vi "37YY250X-1 Phillips DXR.vi"() -> ()   [LabVIEW 2013]
uses:
  <vilib>/Instr/_visa.llb/VISA Configure Serial Port (Instr).vi
panel:
  in  "enumPart":T1(ring)
  in  "Serial Port":refnum<visa-resource-name>
  out "String":string
  out "bDomeClosed":bool
  out "SW VER":string
  out "Employee ID":string
  out "dlbLED":dbl[](array[numeric])
  out "Serial Out 2":i32[](array[numeric])
  out "dlbAllLEDs":dbl
  out "bPassFail":bool
  out "TIMER":dbl
  in  "btnStart":bool
  out "bKeys":bool
  out "bLEDs":bool
  in  "btnExit":bool
  out "Cluster":T2
  out "Serial Out":i32[](array[numeric])
  in  "btnStop":bool
  out "Serial In":u8[](array[numeric])=[165, 1, 31, 32] format="%.0x"
  out "Boolean":bool
  # "Serial Data\nByte 0 Sync\nByte 1 CMD\nByte 2 PORT DATA\nByte 3 BitMask\nByte 4 KeyMap"
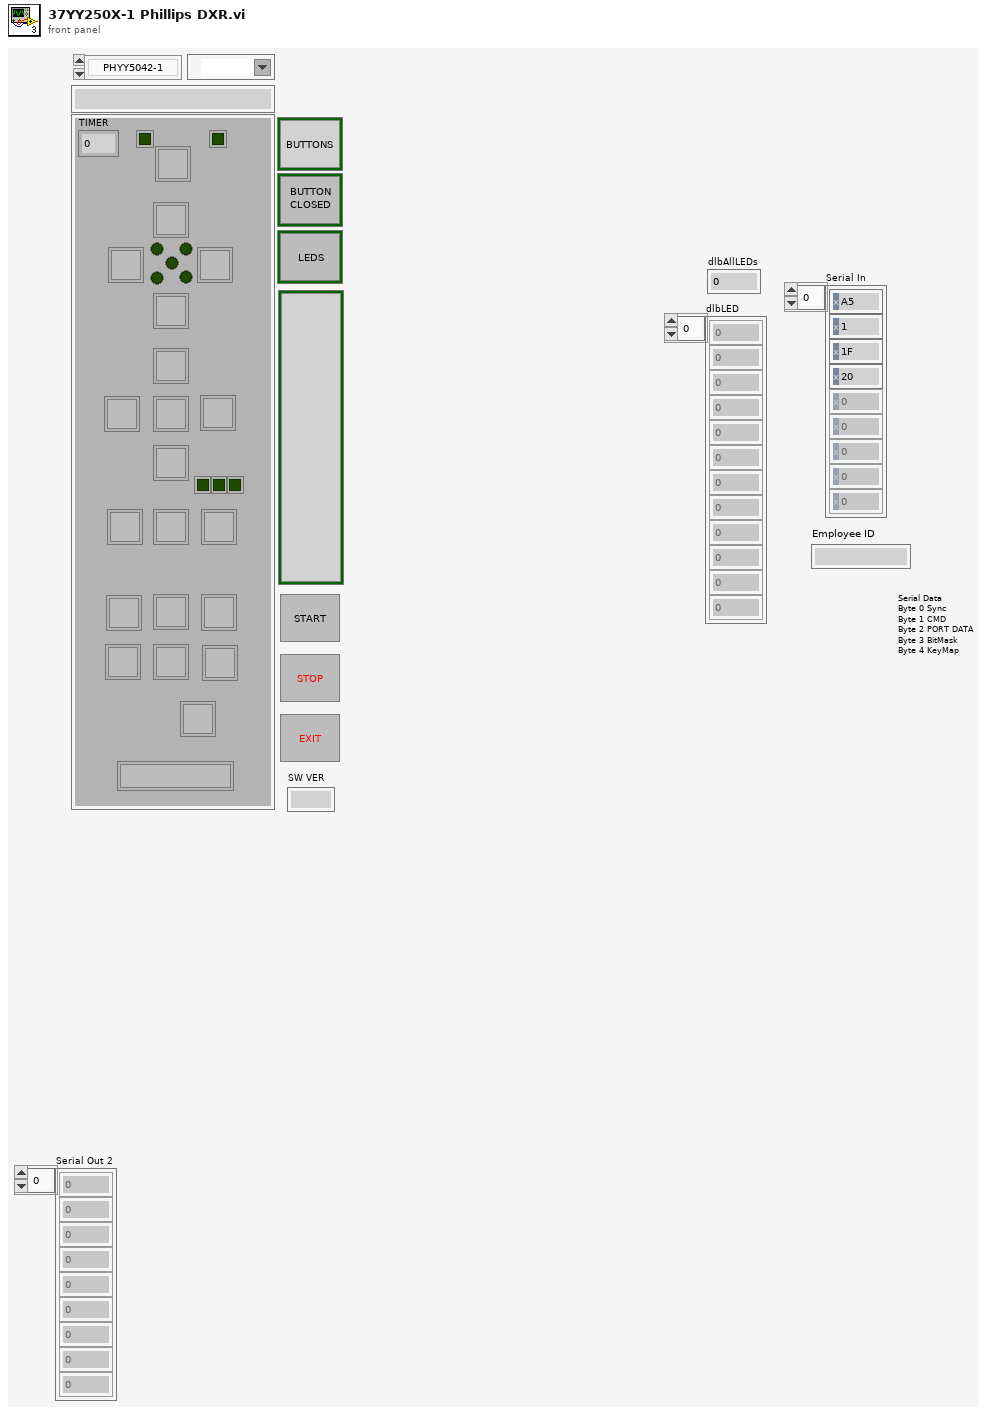
[diagram p1: front panel]
types:
  T1 = enum16{"PHYY5042-1", "PHYY5043-1", "PHYY5037-1", "PHYY5037-2", "PHYY5071-1", "PHYY5071-2", "PHYY5110-1", "PHYY5110-2"}
  T2 = cluster{"bLed 0":bool, "bLed 1":bool, "bLed 2":bool, "bLed 3":bool, "bLed 4":bool, "bLed 5":bool, "bLed 6":bool, "bLed 7":bool, "bLed 8":bool, "bLed 9":bool, "DS 1":bool, "DS 2":bool, "DS 3":bool, "DS 4":bool, "DS 5":bool, "DS 6":bool, "DS 7":bool, "DS 8":bool, "DS 9":bool, "DS 10":bool, "DS 11":bool, "DS 12":bool, "DS 13":bool, "DS 14":bool, "DS 15":bool, "DS 16":bool, "DS 17":bool, "DS 18":bool, "DS 19":bool, "DS 20":bool, "DS 21":bool, "bFalseImage":bool, "bFalseImage 2":bool, "bIcon":bool, "bIcon 2":bool, "Boolean":bool, "Boolean 2":bool, "Boolean 3":bool}
  T3 = enum8{"Enabled", "Disabled", "Disabled and Grayed Out"}
  T4 = cluster{"LOG_DIRECTORY":string, "LOG_FILE":string, "Part Number":string[], "Base Part Number":string[]}
  T5 = enum16{"SET DEFAULTS", "ENABLE POWER", "SCAN FOR CLOSED KEYS", "KEY TEST", "LED TEST", "DISABLE POWER", "TEST END"}
  T6 = cluster{"dlbLED":dbl[], "dlbAllLEDs":dbl, "Pass/Fail":bool, "Keys":bool, "LEDS":bool, "Employee ID":string, "Part Number":string, "SW Version":string}
  T7 = enum32{"invalid app kind", "Development System", "Run Time System", "Student Edition", "Embedded LabVIEW", "Evaluation", "Custom"}
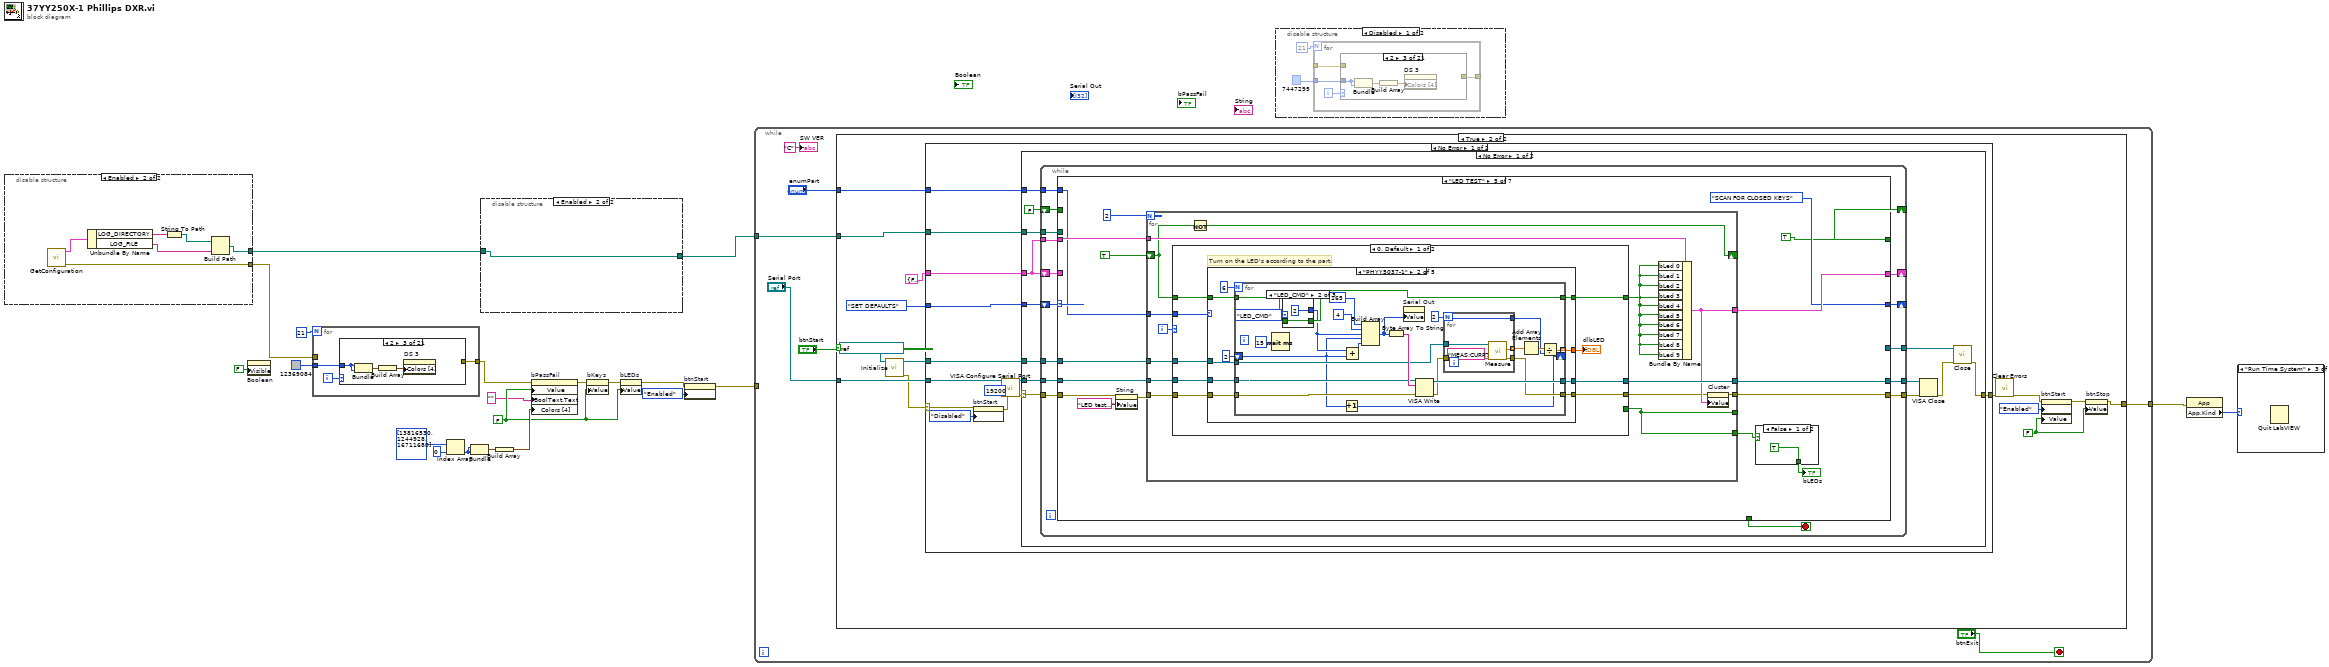
[diagram p0: block diagram]
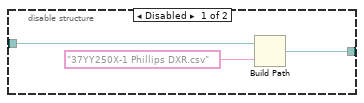
[diagram p8: hidden frame]
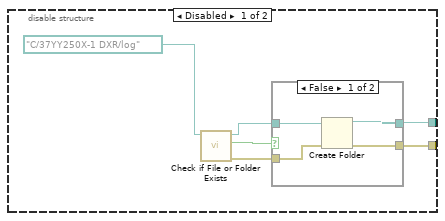
[diagram p9: hidden frame]
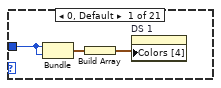
[diagram p11: hidden frame]
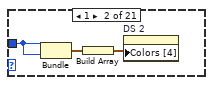
[diagram p12: hidden frame]
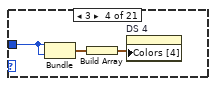
[diagram p13: hidden frame]
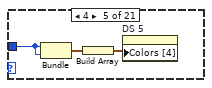
[diagram p14: hidden frame]
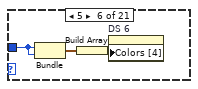
[diagram p15: hidden frame]
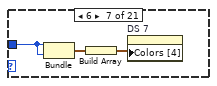
[diagram p16: hidden frame]
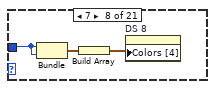
[diagram p17: hidden frame]
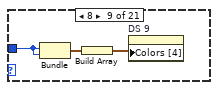
[diagram p18: hidden frame]
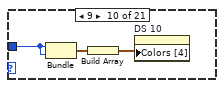
[diagram p19: hidden frame]
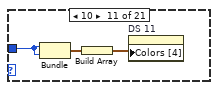
[diagram p20: hidden frame]
diagram:
  w15 = FALSE ("bKeys")
  n1 = disable-structure shown="Enabled" {
    disable-tunnel: [w26 w36] -> w5
    disable-tunnel: [w23 w38] -> w4
    frame Disabled {
      n2 = call <vilib>:"Check if File or Folder Exists.vi"("path"=path "C:/37YY250X-1 DXR/log" ("file path (dialog if empty)")) -> ("error out"=w24:errorcluster, "file or folder exists?"=w27:bool, "dup path"=w25:path)  [unwired: 8 in]
      n3 = case shown="False" w27 {
        tunnel: [w30 w32] -> w26
        tunnel: w25 -> [w31 w32]
        tunnel: w24 -> [w29 _]
        tunnel: [w28 _] -> w23
        frame False {
          n4 = Create Folder(path (use dialog)=w31, error in=w29) -> (created path=w30:path, error out=w28:errorcluster)  [unwired: 1 in, 1 out]
        }
        frame True {
        }
      }
    }
    frame Enabled {
      n5 = call "GetConfiguration.vi"() -> ("error out"=w38:errorcluster, "Cluster"=w37:T4)  [unwired: 9 in, 1 out]
      n6 = Unbundle By Name(w37) -> ("LOG_DIRECTORY"=w35:string, "LOG_FILE"=w33:string)
      n7 = String To Path(string=w35) -> (path=w34:path)
      n8 = Build Path(base path=w34, name or relative path=w33) -> (appended path=w36:path)
    }
  }
  n9 = property on="Boolean" class="Bool (strict)"("Visible"=FALSE) -> ()  [unwired: 2 in, 2 out]
  n10 = for {
    N: 21 -> [_]
    tunnel: u32 12369084 -> [w40]
    tunnel: [w39] -> w7
    tunnel: w4 -> [_]
    i -> [w41]
    n11 = case shown="2" w41 {
      tunnel: w40 -> [w42 w45 w48 w51 w54 w57 w60 w63 w66 w69 w72 w75 w78 w81 w84 w87 w90 w93 w96 w99 w103]
      tunnel: [_ _ _ _ _ _ _ _ _ _ _ _ _ _ _ _ _ _ _ _ w102] -> w39
      frame 0, Default {
        n12 = Bundle(w42, w42) -> (w44:cluster{u32, u32})  [unwired: 1 in]
        n13 = Build Array(w44) -> (w43:cluster{u32, u32}[])
        n14 = property on="DS 1" class="Bool (strict)"("Colors [4]"=w43) -> ()  [unwired: 2 in, 2 out]
      }
      frame 1 {
        n15 = Bundle(w45, w45) -> (w47:cluster{u32, u32})  [unwired: 1 in]
        n16 = Build Array(w47) -> (w46:cluster{u32, u32}[])
        n17 = property on="DS 2" class="Bool (strict)"("Colors [4]"=w46) -> ()  [unwired: 2 in, 2 out]
      }
      frame 2 {
        n18 = Bundle(w48, w48) -> (w50:cluster{u32, u32})  [unwired: 1 in]
        n19 = Build Array(w50) -> (w49:cluster{u32, u32}[])
        n20 = property on="DS 3" class="Bool (strict)"("Colors [4]"=w49) -> ()  [unwired: 2 in, 2 out]
      }
      frame 3 {
        n21 = Bundle(w51, w51) -> (w52:cluster{u32, u32})  [unwired: 1 in]
        n22 = Build Array(w52) -> (w53:cluster{u32, u32}[])
        n23 = property on="DS 4" class="Bool (strict)"("Colors [4]"=w53) -> ()  [unwired: 2 in, 2 out]
      }
      frame 4 {
        n24 = Bundle(w54, w54) -> (w56:cluster{u32, u32})  [unwired: 1 in]
        n25 = Build Array(w56) -> (w55:cluster{u32, u32}[])
        n26 = property on="DS 5" class="Bool (strict)"("Colors [4]"=w55) -> ()  [unwired: 2 in, 2 out]
      }
      frame 5 {
        n27 = Bundle(w57, w57) -> (w59:cluster{u32, u32})  [unwired: 1 in]
        n28 = Build Array(w59) -> (w58:cluster{u32, u32}[])
        n29 = property on="DS 6" class="Bool (strict)"("Colors [4]"=w58) -> ()  [unwired: 2 in, 2 out]
      }
      frame 6 {
        n30 = Bundle(w60, w60) -> (w62:cluster{u32, u32})  [unwired: 1 in]
        n31 = Build Array(w62) -> (w61:cluster{u32, u32}[])
        n32 = property on="DS 7" class="Bool (strict)"("Colors [4]"=w61) -> ()  [unwired: 2 in, 2 out]
      }
      frame 7 {
        n33 = Bundle(w63, w63) -> (w65:cluster{u32, u32})  [unwired: 1 in]
        n34 = Build Array(w65) -> (w64:cluster{u32, u32}[])
        n35 = property on="DS 8" class="Bool (strict)"("Colors [4]"=w64) -> ()  [unwired: 2 in, 2 out]
      }
      frame 8 {
        n36 = Bundle(w66, w66) -> (w68:cluster{u32, u32})  [unwired: 1 in]
        n37 = Build Array(w68) -> (w67:cluster{u32, u32}[])
        n38 = property on="DS 9" class="Bool (strict)"("Colors [4]"=w67) -> ()  [unwired: 2 in, 2 out]
      }
      frame 9 {
        n39 = Bundle(w69, w69) -> (w71:cluster{u32, u32})  [unwired: 1 in]
        n40 = Build Array(w71) -> (w70:cluster{u32, u32}[])
        n41 = property on="DS 10" class="Bool (strict)"("Colors [4]"=w70) -> ()  [unwired: 2 in, 2 out]
      }
      frame 10 {
        n42 = Bundle(w72, w72) -> (w74:cluster{u32, u32})  [unwired: 1 in]
        n43 = Build Array(w74) -> (w73:cluster{u32, u32}[])
        n44 = property on="DS 11" class="Bool (strict)"("Colors [4]"=w73) -> ()  [unwired: 2 in, 2 out]
      }
      frame 11 {
        n45 = Bundle(w75, w75) -> (w76:cluster{u32, u32})  [unwired: 1 in]
        n46 = Build Array(w76) -> (w77:cluster{u32, u32}[])
        n47 = property on="DS 12" class="Bool (strict)"("Colors [4]"=w77) -> ()  [unwired: 2 in, 2 out]
      }
      frame 12 {
        n48 = Bundle(w78, w78) -> (w80:cluster{u32, u32})  [unwired: 1 in]
        n49 = Build Array(w80) -> (w79:cluster{u32, u32}[])
        n50 = property on="DS 13" class="Bool (strict)"("Colors [4]"=w79) -> ()  [unwired: 2 in, 2 out]
      }
      frame 13 {
        n51 = Bundle(w81, w81) -> (w83:cluster{u32, u32})  [unwired: 1 in]
        n52 = Build Array(w83) -> (w82:cluster{u32, u32}[])
        n53 = property on="DS 14" class="Bool (strict)"("Colors [4]"=w82) -> ()  [unwired: 2 in, 2 out]
      }
      frame 14 {
        n54 = Bundle(w84, w84) -> (w86:cluster{u32, u32})  [unwired: 1 in]
        n55 = Build Array(w86) -> (w85:cluster{u32, u32}[])
        n56 = property on="DS 15" class="Bool (strict)"("Colors [4]"=w85) -> ()  [unwired: 2 in, 2 out]
      }
      frame 15 {
        n57 = Bundle(w87, w87) -> (w89:cluster{u32, u32})  [unwired: 1 in]
        n58 = Build Array(w89) -> (w88:cluster{u32, u32}[])
        n59 = property on="DS 16" class="Bool (strict)"("Colors [4]"=w88) -> ()  [unwired: 2 in, 2 out]
      }
      frame 16 {
        n60 = Bundle(w90, w90) -> (w92:cluster{u32, u32})  [unwired: 1 in]
        n61 = Build Array(w92) -> (w91:cluster{u32, u32}[])
        n62 = property on="DS 17" class="Bool (strict)"("Colors [4]"=w91) -> ()  [unwired: 2 in, 2 out]
      }
      frame 17 {
        n63 = Bundle(w93, w93) -> (w95:cluster{u32, u32})  [unwired: 1 in]
        n64 = Build Array(w95) -> (w94:cluster{u32, u32}[])
        n65 = property on="DS 18" class="Bool (strict)"("Colors [4]"=w94) -> ()  [unwired: 2 in, 2 out]
      }
      frame 18 {
        n66 = Bundle(w96, w96) -> (w98:cluster{u32, u32})  [unwired: 1 in]
        n67 = Build Array(w98) -> (w97:cluster{u32, u32}[])
        n68 = property on="DS 19" class="Bool (strict)"("Colors [4]"=w97) -> ()  [unwired: 2 in, 2 out]
      }
      frame 19 {
        n69 = Bundle(w99, w99) -> (w101:cluster{u32, u32})  [unwired: 1 in]
        n70 = Build Array(w101) -> (w100:cluster{u32, u32}[])
        n71 = property on="DS 20" class="Bool (strict)"("Colors [4]"=w100) -> ()  [unwired: 2 in, 2 out]
      }
      frame 20 {
        n72 = Bundle(w103, w103) -> (w105:cluster{u32, u32})  [unwired: 1 in]
        n73 = Build Array(w105) -> (w104:cluster{u32, u32}[])
        n74 = property on="DS 21" class="Bool (strict)"("Colors [4]"=w104) -> (error out=w102:errorcluster)  [unwired: 2 in, 1 out]
      }
    }
  }
  n75 = Index Array(array=u32[] [13816530, 1244928, 16711680], index=0) -> (element=w18:u32)
  n76 = Bundle(w18, w18) -> (w19:cluster{u32, u32})  [unwired: 1 in]
  n77 = disable-structure shown="Enabled" {
    disable-tunnel: [w107 w109] -> w6
    disable-tunnel: w5 -> [w106 w109]
    frame Disabled {
      n78 = Build Path(base path=w106, name or relative path="37YY250X-1 Phillips DXR.csv") -> (appended path=w107:path)
    }
    frame Enabled {
    }
  }
  n79 = Build Array(w19) -> (w20:cluster{u32, u32}[])
  n80 = property on="bPassFail" class="Bool (strict)"(error in=w7, "Value"=w15, "BoolText.Text"="" ("Boolean Text.Text"), "Colors [4]"=w20) -> (error out=w13:errorcluster)  [unwired: 1 in, 1 out]
  n81 = property on="bKeys" class="Bool (strict)"(error in=w13, "Value"=w15) -> (error out=w12:errorcluster)  [unwired: 1 in, 1 out]
  n82 = property on="bLEDs" class="Bool (strict)"(error in=w12, "Value"=w15) -> (error out=w11:errorcluster)  [unwired: 1 in, 1 out]
  n83 = property on="btnStart" class="Bool (strict)"(error in=w11, "DisabledEnum"=T3."Enabled" ("Disabled")) -> (error out=w10:errorcluster)  [unwired: 1 in, 1 out]
  n84 = while {
    tunnel: [w115] -> w2
    tunnel: w10 -> [_]
    tunnel: w6 -> [w112]
    stop <- "btnExit" stop-if-true
    n85 = case shown="True" "btnStart" {
      tunnel: [_ w196] -> w115
      tunnel: w112 -> [w143 w192]
      tunnel: "Serial Port" -> [_ w191]
      tunnel: "enumPart" -> [w119 w189]
      frame False {
        n86 = case shown="\"PHYY5110-2\"" w119 {
          tunnel: [w148 w150 w152 w154 w155 w162 w174] -> w137
          tunnel: [w148 w150 w152 w154 w155 w163 w175] -> w136
          tunnel: [w148 w150 w152 w154 w155 w161 w173] -> w135
          tunnel: [w148 w150 w152 w154 w155 w164 w176] -> w134
          tunnel: [w148 w150 w152 w154 w155 w165 w177] -> w133
          tunnel: [w148 w150 w152 w154 w155 w166 w178] -> w132
          tunnel: [w148 w150 w152 w154 w155 w167 w179] -> w131
          tunnel: [w148 w150 w152 w154 w155 w158 w170] -> w130
          tunnel: [w148 w150 w152 w154 w155 w159 w171] -> w129
          tunnel: [w148 w150 w152 w154 w155 w159 w171] -> w128
          tunnel: [w148 w150 w152 w154 w155 w159 w171] -> w127
          tunnel: [w148 w150 w152 w154 w155 w159 w171] -> w126
          tunnel: [w148 _ _ _ _ w160 w172] -> w125
          tunnel: [w148 _ _ _ _ w160 w172] -> w124
          tunnel: [w148 _ _ _ _ w160 w172] -> w123
          tunnel: [w148 _ _ _ _ _ _] -> w122
          tunnel: [w148 w150 w152 w154 w155 w168 w180] -> w121
          tunnel: [FALSE TRUE TRUE w154 TRUE w160 w172] -> w120
          tunnel: [w148 w150 w152 w154 w155 w159 w171] -> w118
          tunnel: [_ _ _ _ _ TRUE TRUE] -> w117
          frame "PHYY5042-1", Default {
            w148 = TRUE
          }
          frame "PHYY5037-1" {
            w150 = FALSE
          }
          frame "PHYY5071-1" {
            w152 = FALSE
          }
          frame "PHYY5071-2" {
            w154 = TRUE
          }
          frame "PHYY5037-2" {
            w155 = FALSE
          }
          frame "PHYY5110-1" {
            w160 = FALSE
            w159 = TRUE
            n87 = Not(x=w159) -> (.not. x?=w158:bool)
            n88 = Not(x=w159) -> (.not. x?=w162:bool)
            n89 = Not(x=w159) -> (.not. x?=w163:bool)
            n90 = Not(x=w159) -> (.not. x?=w161:bool)
            n91 = Not(x=w159) -> (.not. x?=w164:bool)
            n92 = Not(x=w159) -> (.not. x?=w165:bool)
            n93 = Not(x=w159) -> (.not. x?=w166:bool)
            n94 = Not(x=w159) -> (.not. x?=w167:bool)
            n95 = Not(x=w159) -> (.not. x?=w168:bool)
          }
          frame "PHYY5110-2" {
            w172 = FALSE
            w171 = TRUE
            n96 = Not(x=w171) -> (.not. x?=w170:bool)
            n97 = Not(x=w171) -> (.not. x?=w174:bool)
            n98 = Not(x=w171) -> (.not. x?=w175:bool)
            n99 = Not(x=w171) -> (.not. x?=w173:bool)
            n100 = Not(x=w171) -> (.not. x?=w176:bool)
            n101 = Not(x=w171) -> (.not. x?=w177:bool)
            n102 = Not(x=w171) -> (.not. x?=w178:bool)
            n103 = Not(x=w171) -> (.not. x?=w179:bool)
            n104 = Not(x=w171) -> (.not. x?=w180:bool)
          }
        }
        n105 = property on="DS 15" class="Bool (strict)"("Visible"=w137) -> ()  [unwired: 2 in, 2 out]
        n106 = property on="DS 12" class="Bool (strict)"("Visible"=w136) -> ()  [unwired: 2 in, 2 out]
        n107 = property on="DS 14" class="Bool (strict)"("Visible"=w134) -> ()  [unwired: 2 in, 2 out]
        n108 = property on="DS 13" class="Bool (strict)"("Visible"=w135) -> ()  [unwired: 2 in, 2 out]
        n109 = property on="DS 8" class="Bool (strict)"("Visible"=w132) -> ()  [unwired: 2 in, 2 out]
        n110 = property on="DS 9" class="Bool (strict)"("Visible"=w131) -> ()  [unwired: 2 in, 2 out]
        n111 = property on="DS 11" class="Bool (strict)"("Visible"=w133) -> ()  [unwired: 2 in, 2 out]
        n112 = property on="DS 5" class="Bool (strict)"("Visible"=w129) -> ()  [unwired: 2 in, 2 out]
        n113 = property on="DS 10" class="Bool (strict)"("Visible"=w130) -> ()  [unwired: 2 in, 2 out]
        n114 = property on="DS 2" class="Bool (strict)"("Visible"=w128) -> ()  [unwired: 2 in, 2 out]
        n115 = property on="DS 7" class="Bool (strict)"("Visible"=w127) -> ()  [unwired: 2 in, 2 out]
        n116 = property on="DS 4" class="Bool (strict)"("Visible"=w126) -> ()  [unwired: 2 in, 2 out]
        n117 = property on="DS 1" class="Bool (strict)"("Visible"=w121) -> ()  [unwired: 2 in, 2 out]
        n118 = property on="DS 3" class="Bool (strict)"("Visible"=w118) -> ()  [unwired: 2 in, 2 out]
        n119 = property on="bFalseImage" class="Bool (strict)"("Visible"=w120) -> ()  [unwired: 2 in, 2 out]
        n120 = property on="bLed 1" class="Bool (strict)"("Visible"=w125) -> ()  [unwired: 2 in, 2 out]
        n121 = property on="bLed 7" class="Bool (strict)"("Visible"=w124) -> ()  [unwired: 2 in, 2 out]
        n122 = property on="bFalseImage 2" class="Bool (strict)"("Visible"=w120) -> ()  [unwired: 2 in, 2 out]
        n123 = property on="bLed 9" class="Bool (strict)"("Visible"=w122) -> ()  [unwired: 2 in, 2 out]
        n124 = property on="bLed 8" class="Bool (strict)"("Visible"=w123) -> ()  [unwired: 2 in, 2 out]
        n125 = property on="bIcon" class="Bool (strict)"("Visible"=w120) -> ()  [unwired: 2 in, 2 out]
        n126 = property on="bIcon 2" class="Bool (strict)"("Visible"=w120) -> ()  [unwired: 2 in, 2 out]
        n127 = property on="Boolean" class="Bool (strict)"("Visible"=w117) -> ()  [unwired: 2 in, 2 out]
        n128 = property on="Boolean 3" class="Bool (strict)"("Visible"=w117) -> ()  [unwired: 2 in, 2 out]
        n129 = property on="Boolean 2" class="Bool (strict)"("Visible"=w117) -> ()  [unwired: 2 in, 2 out]
        n130 = property on="btnStop" class="Bool (strict)"("Value"=FALSE ("btnStop")) -> (error out=w140:errorcluster)  [unwired: 2 in, 1 out]
        n131 = property on="String" class="Str"(error in=w140, "Value"="Press start..." ("String")) -> (error out=w139:errorcluster)  [unwired: 1 in, 1 out]
        n132 = First Call?() -> (First Call?: T/F=w146:bool)
        n133 = case shown="False" w146 {
          tunnel: w139 -> [w186 _]
          tunnel: [w186 _] -> w138
          frame False {
          }
          frame True {
            n134 = call "Get Operator ID.vi"() -> ("Employee ID"=→"Employee ID":string)
          }
        }
        n135 = Current VI's Menubar() -> (w145:refnum<k9>)
        n136 = Get Menu Selection(0:w145, 3:w138) -> (6:w144:string)  [unwired: 2 in, 4 out]
        n137 = call <vilib>:"Trim Whitespace.vi"("string"=w144) -> ("trimmed string"=w142:string)  [unwired: 1 in]
        n138 = case shown="\"Log File Location_1\"" w142 {
          tunnel: w143 -> [_ w185 _]
          frame "False", Default {
          }
          frame "Log File Location_1" {
            n139 = Path To String(path=w185) -> (string=w184:string)
            n140 = call <vilib>:"Space Constant.vi"() -> ("String"=w181:string)
            n141 = Concatenate Strings("Log File Location:" ("string"), w181, w184) -> (w183:string)
            n142 = One Button Dialog(message=w183) -> ()  [unwired: 1 in, 1 out]
          }
          frame "Serial Port" {
          }
        }
      }
      frame True {
        w197 = FALSE ("btnStart")
        n143 = call <instrlib>:"Initialize.vi"("VISA resource name"=refnum<visa-resource-name> "GPIB0::5::INSTR" ("Instrument Resource Name")) -> ("error out"=w190:errorcluster, "VISA resource name out"=w194:refnum<visa-resource-name>)  [unwired: 9 in]
        n144 = case shown="No Error" w190 {
          selector: w190 -> [w203 w1027]
          tunnel: [w214 _] -> w200
          tunnel: T5."SET DEFAULTS" -> [w211 _]
          tunnel: T2 {"bLed 0"=FALSE, "bLed 1"=FALSE, "bLed 2"=FALSE, "bLed 3"=FALSE, "bLed 4"=FALSE, "bLed 5"=FALSE, "bLed 6"=FALSE, "bLed 7"=FALSE, "bLed 8"=FALSE, "bLed 9"=FALSE, "DS 1"=FALSE, "DS 2"=FALSE, "DS 3"=FALSE, "DS 4"=FALSE, "DS 5"=FALSE, "DS 6"=FALSE, "DS 7"=FALSE, "DS 8"=FALSE, "DS 9"=FALSE, "DS 10"=FALSE, "DS 11"=FALSE, "DS 12"=FALSE, "DS 13"=FALSE, "DS 14"=FALSE, "DS 15"=FALSE, "DS 16"=FALSE, "DS 17"=FALSE, "DS 18"=FALSE, "DS 19"=FALSE, "DS 20"=FALSE, "DS 21"=FALSE, "bFalseImage"=FALSE, "bFalseImage 2"=FALSE, "bIcon"=FALSE, "bIcon 2"=FALSE, "Boolean"=FALSE, "Boolean 2"=FALSE, "Boolean 3"=FALSE} ("Cluster 2") -> [w210 _]
          tunnel: w194 -> [w207 _]
          tunnel: w192 -> [w205 _]
          tunnel: w191 -> [w204 _]
          tunnel: w189 -> [w202 _]
          frame No Error {
            n145 = property on="btnStart" class="Bool (strict)"(error in=w203, "DisabledEnum"=T3."Disabled" ("Disabled")) -> (error out=w209:errorcluster)  [unwired: 1 in, 1 out]
            n146 = call-poly "VISA Configure Serial Port"("VISA resource name"=w204, "baud rate (9600)"=u32 19200, "error in (no error)"=w209) -> ("VISA resource name out"=w213:refnum<visa-resource-name>, "error out"=w206:errorcluster)  [unwired: 11 in]
            n147 = case shown="No Error" w206 {
              selector: w206 -> [w222 w1021]
              tunnel: w213 -> [w227 _]
              tunnel: w211 -> [w224 _]
              tunnel: w210 -> [w223 _]
              tunnel: [w219 _] -> w214
              tunnel: w207 -> [w221 _]
              tunnel: w205 -> [w217 _]
              tunnel: w202 -> [w215 _]
              frame No Error {
                n148 = while {
                  tunnel: w227 -> [w243]
                  tunnel: w222 -> [w242]
                  tunnel: [w241] -> w226
                  tunnel: [w240] -> w225
                  shift-right: [w236] -> _
                  shift-left: w224 -> [w237]
                  shift-right: [w239] -> _
                  shift-left: w223 -> [w238]
                  tunnel: w223 -> [w234]
                  tunnel: w221 -> [w233]
                  tunnel: [w232] -> w218
                  tunnel: w217 -> [w231]
                  shift-right: [w230] -> _
                  shift-left: FALSE -> [w229]
                  tunnel: w215 -> [w228]
                  stop <- w235 stop-if-true
                  n149 = case shown="\"LED TEST\"" w237 {
                    tunnel: w243 -> [w262 _ w357 w384 w669 _ w1005]
                    tunnel: w242 -> [w245 w333 w349 w373 w658 w956 w979]
                    tunnel: [w262 _ w355 w383 w668 _ w1005] -> w241
                    tunnel: [w248 w336 w356 w382 w666 w960 w975] -> w240
                    tunnel: [_ _ _ w381 w667 w963 w1004] -> w239
                    tunnel: w238 -> [_ _ _ w380 _ w963 w1004]
                    tunnel: [T5."ENABLE POWER" w331 w358 w378 T5."SCAN FOR CLOSED KEYS" T5."TEST END" _] -> w236
                    tunnel: [_ _ _ _ _ _ TRUE] -> w235
                    tunnel: w234 -> [_ _ _ _ w663 _ _]
                    tunnel: w233 -> [_ w339 _ _ w662 w962 _]
                    tunnel: [_ _ _ _ _ w959 _] -> w232
                    tunnel: w231 -> [_ _ _ _ _ _ w981]
                    tunnel: [_ _ _ _ TRUE _ _] -> w230
                    tunnel: w229 -> [_ _ w351 _ _ _ _]
                    tunnel: w228 -> [_ _ _ w370 w654 _ _]
                    frame "SET DEFAULTS", Default {
                      w247 = FALSE ("bKeys")
                      n150 = property on="String" class="Str"(error in=w245, "Value"="Set defaults..." ("String")) -> (error out=w246:errorcluster)  [unwired: 1 in, 1 out]
                      n151 = for {
                        N: 21 -> [_]
                        tunnel: u32 12369084 -> [w265]
                        tunnel: [w264] -> w251
                        tunnel: w246 -> [w263]
                        i -> [w266]
                        n152 = case shown="2" w266 {
                          tunnel: w265 -> [w267 w270 w273 w276 w279 w282 w285 w288 w291 w294 w297 w300 w303 w306 w309 w312 w315 w318 w321 w324 w328]
                          tunnel: [_ _ _ _ _ _ _ _ _ _ _ _ _ _ _ _ _ _ _ _ w327] -> w264
                          tunnel: w263 -> [_ _ _ _ _ _ _ _ _ _ _ _ _ _ _ _ _ _ _ _ _]
                          frame 0, Default {
                            n153 = Bundle(w267, w267) -> (w269:cluster{u32, u32})  [unwired: 1 in]
                            n154 = Build Array(w269) -> (w268:cluster{u32, u32}[])
                            n155 = property on="DS 1" class="Bool (strict)"("Colors [4]"=w268) -> ()  [unwired: 2 in, 2 out]
                          }
                          frame 1 {
                            n156 = Bundle(w270, w270) -> (w272:cluster{u32, u32})  [unwired: 1 in]
                            n157 = Build Array(w272) -> (w271:cluster{u32, u32}[])
                            n158 = property on="DS 2" class="Bool (strict)"("Colors [4]"=w271) -> ()  [unwired: 2 in, 2 out]
                          }
                          frame 2 {
                            n159 = Bundle(w273, w273) -> (w275:cluster{u32, u32})  [unwired: 1 in]
                            n160 = Build Array(w275) -> (w274:cluster{u32, u32}[])
                            n161 = property on="DS 3" class="Bool (strict)"("Colors [4]"=w274) -> ()  [unwired: 2 in, 2 out]
                          }
                          frame 3 {
                            n162 = Bundle(w276, w276) -> (w277:cluster{u32, u32})  [unwired: 1 in]
                            n163 = Build Array(w277) -> (w278:cluster{u32, u32}[])
                            n164 = property on="DS 4" class="Bool (strict)"("Colors [4]"=w278) -> ()  [unwired: 2 in, 2 out]
                          }
                          frame 4 {
                            n165 = Bundle(w279, w279) -> (w281:cluster{u32, u32})  [unwired: 1 in]
                            n166 = Build Array(w281) -> (w280:cluster{u32, u32}[])
                            n167 = property on="DS 5" class="Bool (strict)"("Colors [4]"=w280) -> ()  [unwired: 2 in, 2 out]
                          }
                          frame 5 {
                            n168 = Bundle(w282, w282) -> (w284:cluster{u32, u32})  [unwired: 1 in]
                            n169 = Build Array(w284) -> (w283:cluster{u32, u32}[])
                            n170 = property on="DS 6" class="Bool (strict)"("Colors [4]"=w283) -> ()  [unwired: 2 in, 2 out]
                          }
                          frame 6 {
                            n171 = Bundle(w285, w285) -> (w287:cluster{u32, u32})  [unwired: 1 in]
                            n172 = Build Array(w287) -> (w286:cluster{u32, u32}[])
                            n173 = property on="DS 7" class="Bool (strict)"("Colors [4]"=w286) -> ()  [unwired: 2 in, 2 out]
                          }
                          frame 7 {
                            n174 = Bundle(w288, w288) -> (w290:cluster{u32, u32})  [unwired: 1 in]
                            n175 = Build Array(w290) -> (w289:cluster{u32, u32}[])
                            n176 = property on="DS 8" class="Bool (strict)"("Colors [4]"=w289) -> ()  [unwired: 2 in, 2 out]
                          }
                          frame 8 {
                            n177 = Bundle(w291, w291) -> (w293:cluster{u32, u32})  [unwired: 1 in]
                            n178 = Build Array(w293) -> (w292:cluster{u32, u32}[])
                            n179 = property on="DS 9" class="Bool (strict)"("Colors [4]"=w292) -> ()  [unwired: 2 in, 2 out]
                          }
                          frame 9 {
                            n180 = Bundle(w294, w294) -> (w296:cluster{u32, u32})  [unwired: 1 in]
                            n181 = Build Array(w296) -> (w295:cluster{u32, u32}[])
                            n182 = property on="DS 10" class="Bool (strict)"("Colors [4]"=w295) -> ()  [unwired: 2 in, 2 out]
                          }
                          frame 10 {
                            n183 = Bundle(w297, w297) -> (w299:cluster{u32, u32})  [unwired: 1 in]
                            n184 = Build Array(w299) -> (w298:cluster{u32, u32}[])
                            n185 = property on="DS 11" class="Bool (strict)"("Colors [4]"=w298) -> ()  [unwired: 2 in, 2 out]
                          }
                          frame 11 {
                            n186 = Bundle(w300, w300) -> (w301:cluster{u32, u32})  [unwired: 1 in]
                            n187 = Build Array(w301) -> (w302:cluster{u32, u32}[])
                            n188 = property on="DS 12" class="Bool (strict)"("Colors [4]"=w302) -> ()  [unwired: 2 in, 2 out]
                          }
                          frame 12 {
                            n189 = Bundle(w303, w303) -> (w305:cluster{u32, u32})  [unwired: 1 in]
                            n190 = Build Array(w305) -> (w304:cluster{u32, u32}[])
                            n191 = property on="DS 13" class="Bool (strict)"("Colors [4]"=w304) -> ()  [unwired: 2 in, 2 out]
                          }
                          frame 13 {
                            n192 = Bundle(w306, w306) -> (w308:cluster{u32, u32})  [unwired: 1 in]
                            n193 = Build Array(w308) -> (w307:cluster{u32, u32}[])
                            n194 = property on="DS 14" class="Bool (strict)"("Colors [4]"=w307) -> ()  [unwired: 2 in, 2 out]
                          }
                          frame 14 {
                            n195 = Bundle(w309, w309) -> (w311:cluster{u32, u32})  [unwired: 1 in]
                            n196 = Build Array(w311) -> (w310:cluster{u32, u32}[])
                            n197 = property on="DS 15" class="Bool (strict)"("Colors [4]"=w310) -> ()  [unwired: 2 in, 2 out]
                          }
                          frame 15 {
                            n198 = Bundle(w312, w312) -> (w314:cluster{u32, u32})  [unwired: 1 in]
                            n199 = Build Array(w314) -> (w313:cluster{u32, u32}[])
                            n200 = property on="DS 16" class="Bool (strict)"("Colors [4]"=w313) -> ()  [unwired: 2 in, 2 out]
                          }
                          frame 16 {
                            n201 = Bundle(w315, w315) -> (w317:cluster{u32, u32})  [unwired: 1 in]
                            n202 = Build Array(w317) -> (w316:cluster{u32, u32}[])
                            n203 = property on="DS 17" class="Bool (strict)"("Colors [4]"=w316) -> ()  [unwired: 2 in, 2 out]
                          }
                          frame 17 {
                            n204 = Bundle(w318, w318) -> (w320:cluster{u32, u32})  [unwired: 1 in]
                            n205 = Build Array(w320) -> (w319:cluster{u32, u32}[])
                            n206 = property on="DS 18" class="Bool (strict)"("Colors [4]"=w319) -> ()  [unwired: 2 in, 2 out]
                          }
                          frame 18 {
                            n207 = Bundle(w321, w321) -> (w323:cluster{u32, u32})  [unwired: 1 in]
                            n208 = Build Array(w323) -> (w322:cluster{u32, u32}[])
                            n209 = property on="DS 19" class="Bool (strict)"("Colors [4]"=w322) -> ()  [unwired: 2 in, 2 out]
                          }
                          frame 19 {
                            n210 = Bundle(w324, w324) -> (w326:cluster{u32, u32})  [unwired: 1 in]
                            n211 = Build Array(w326) -> (w325:cluster{u32, u32}[])
                            n212 = property on="DS 20" class="Bool (strict)"("Colors [4]"=w325) -> ()  [unwired: 2 in, 2 out]
                          }
                          frame 20 {
                            n213 = Bundle(w328, w328) -> (w330:cluster{u32, u32})  [unwired: 1 in]
                            n214 = Build Array(w330) -> (w329:cluster{u32, u32}[])
                            n215 = property on="DS 21" class="Bool (strict)"("Colors [4]"=w329) -> (error out=w327:errorcluster)  [unwired: 2 in, 1 out]
                          }
                        }
                      }
                      n216 = Index Array(array=u32[] [13816530, 1244928, 16711680], index=0) -> (element=w256:u32)
                      n217 = Bundle(w256, w256) -> (w255:cluster{u32, u32})  [unwired: 1 in]
                      n218 = Build Array(w255) -> (w254:cluster{u32, u32}[])
                      n219 = property on="bPassFail" class="Bool (strict)"(error in=w251, "Value"=w247, "BoolText.Text"="" ("Boolean Text.Text"), "Colors [4]"=w254) -> (error out=w260:errorcluster)  [unwired: 1 in, 1 out]
                      n220 = property on="bKeys" class="Bool (strict)"(error in=w260, "Value"=w247) -> (error out=w261:errorcluster)  [unwired: 1 in, 1 out]
                      n221 = property on="bLEDs" class="Bool (strict)"(error in=w261, "Value"=w247) -> (error out=w249:errorcluster)  [unwired: 1 in, 1 out]
                      n222 = property on="bDomeClosed" class="Bool (strict)"(error in=w249, "Value"=w247) -> (error out=w248:errorcluster)  [unwired: 1 in, 1 out]
                    }
                    frame "ENABLE POWER" {
                      n223 = property on="String" class="Str"(error in=w333, "Value"="Enable power..." ("String")) -> (error out=w332:errorcluster)  [unwired: 1 in, 1 out]
                      n224 = call <instrlib>:"Configure Current Limit.vi"("error in (no error)"=w332, "Current Limit (0.0 Amps)"=0.5, "VISA resource name"=w339) -> ("error out"=w344:errorcluster, "VISA resource name out"=w343:refnum<visa-resource-name>)  [unwired: 7 in]
                      n225 = call <instrlib>:"Configure Voltage Level.vi"("error in (no error)"=w344, "Level (0.0 Volts)"=5.0, "VISA resource name"=w343) -> ("error out"=w342:errorcluster, "VISA resource name out"=w341:refnum<visa-resource-name>)  [unwired: 7 in]
                      n226 = call <instrlib>:"Configure Output Enabled.vi"("error in (no error)"=w342, "Output Enabled (F: Off)"=TRUE, "VISA resource name"=w341) -> ("error out"=w335:errorcluster)  [unwired: 7 in, 1 out]
                      n227 = stacked-sequence {
                        tunnel: [w345 _ _] -> w336
                        tunnel: w335 -> [w345 _ _]
                        tunnel: [_ _ T5."SCAN FOR CLOSED KEYS"] -> w331
                        frame #0 {
                        }
                        frame #1 {
                          n228 = Wait (ms)(milliseconds to wait=u32 1000) -> ()  [unwired: 1 out]
                        }
                        frame #2 {
                        }
                      }
                    }
                    frame "SCAN FOR CLOSED KEYS" {
                      n229 = property on="String" class="Str"(error in=w349, "Value"="Check for closed keys..." ("String")) -> (error out=w348:errorcluster)  [unwired: 1 in, 1 out]
                      n230 = for {
                        N: 10 -> [_]
                        tunnel: w348 -> [w369]
                        tunnel: w357 -> [w368]
                        tunnel: [w367] -> w356
                        tunnel: [w366] -> w355
                        tunnel: [w365] -> w353 mode=indexing
                        n231 = Wait (ms)(milliseconds to wait=u32 50) -> ()  [unwired: 1 out]
                        n232 = call "Scan For Closed Key.vi"("error in (no error)"=w369, "VISA Refnum in"=w368) -> ("error out"=w367:errorcluster, "Pass"=w365:bool, "VISA Refnum out"=w366:refnum<visa-resource-name>)  [unwired: 6 in, 1 out]
                      }
                      n233 = Or Array Elements(Boolean array=w353) -> (logical OR=w352:bool)
                      n234 = case shown="False" w351 {
                        tunnel: [w360 T5."DISABLE POWER"] -> w358
                        tunnel: w352 -> [w359 _]
                        frame False {
                          n235 = case shown="False" w359 {
                            tunnel: [T5."KEY TEST" T5."DISABLE POWER"] -> w360
                            frame False {
                            }
                            frame True {
                            }
                          }
                          "bDomeClosed" <- w359
                        }
                        frame True {
                        }
                      }
                    }
                    frame "KEY TEST" {
                      n236 = Get Date/Time In Seconds() -> (seconds since 1Jan1904=w377:timestamp)
                      n237 = property on="String" class="Str"(error in=w373, "Value"="Key test..." ("String")) -> (error out=w374:errorcluster)  [unwired: 1 in, 1 out]
                      n238 = while {
                        tunnel: w384 -> [w406]
                        tunnel: [w405] -> w383
                        tunnel: [w404] -> w382
                        tunnel: w374 -> [w403]
                        shift-right: [w399] -> w381
                        shift-left: w380 -> [w398]
                        shift-right: [w396] -> _
                        shift-left: 1 ("y") -> [w397]
                        tunnel: [w389] -> w378
                        tunnel: w377 -> [w394]
                        tunnel: 30.0 ("Time Target (s)") -> [w393]
                        tunnel: [w388] -> _
                        tunnel: [w387] -> w372
                        tunnel: w370 -> [w386]
                        stop <- w395 stop-if-true
                        n239 = call "Elapsed Time.vi"("seconds since 1Jan1904"=w394, "Time Target (s)"=w393) -> ("Time Remaining"=w392:dbl)  [unwired: 6 in, 1 out]
                        "TIMER" <- w392
                        n240 = Quotient & Remainder(x=w397, y=1000) -> (x-y*floor(x/y)=w401:i32)  [unwired: 1 out]
                        n241 = Equal To 0?(x=w401) -> (x = 0?=w400:bool)
                        n242 = case shown="False" w400 {
                          tunnel: w406 -> [w410 w498]
                          tunnel: [w410 w493] -> w405
                          tunnel: [w411 w492] -> w404
                          tunnel: w403 -> [w411 w488]
                          tunnel: [w413 w491] -> w399
                          tunnel: w398 -> [w413 w490]
                          tunnel: w397 -> [w415 _]
                          tunnel: [w414 1] -> w396
                          tunnel: [w412 _] -> w388
                          tunnel: [w412 _] -> w387
                          tunnel: w386 -> [w409 _]
                          frame False {
                            n243 = Increment(x=w415) -> (x+1=w414:i32)
                            n244 = case shown="\"PHYY5071-2\"" w409 {
                              tunnel: w413 -> [w438 w448 w458 w472 w486]
                              tunnel: [w437 w447 w457 w471 w485] -> w412
                              frame "PHYY5042-1", Default {
                                n245 = Unbundle By Name(w438) -> ("DS 1"=w436:bool, "DS 2"=w435:bool, "DS 3"=w434:bool, "DS 4"=w433:bool, "DS 5"=w432:bool, "DS 6"=w431:bool, "DS 7"=w430:bool, "DS 8"=w429:bool, "DS 9"=w428:bool, "DS 10"=w427:bool, "DS 11"=w426:bool, "DS 12"=w425:bool, "DS 13"=w424:bool, "DS 14"=w423:bool, "DS 15"=w422:bool, "DS 16"=w421:bool, "DS 17"=w420:bool, "DS 18"=w419:bool, "DS 19"=w418:bool, "DS 20"=w417:bool, "DS 21"=w416:bool)
                                n246 = Compound Arithmetic op=AND(w436, w435, w434, w433, w432, w431, w430, w429, w428, w427, w426, w425, w424, w423, w422, w421, w420, w419, w418, w417, w416) -> (w437:bool)
                              }
                              frame "PHYY5037-1" {
                                n247 = Unbundle By Name(w448) -> ("DS 3"=w440:bool, "DS 6"=w439:bool, "DS 16"=w446:bool, "DS 17"=w445:bool, "DS 18"=w444:bool, "DS 19"=w443:bool, "DS 20"=w442:bool, "DS 21"=w441:bool)
                                n248 = Compound Arithmetic op=AND(w440, w439, w446, w445, w444, w443, w442, w441) -> (w447:bool)
                              }
                              frame "PHYY5037-2" {
                                n249 = Unbundle By Name(w458) -> ("DS 3"=w450:bool, "DS 6"=w449:bool, "DS 16"=w456:bool, "DS 17"=w455:bool, "DS 18"=w454:bool, "DS 19"=w453:bool, "DS 20"=w452:bool, "DS 21"=w451:bool)
                                n250 = Compound Arithmetic op=AND(w450, w449, w456, w455, w454, w453, w452, w451) -> (w457:bool)
                              }
                              frame "PHYY5071-1" {
                                n251 = Unbundle By Name(w472) -> ("DS 2"=w464:bool, "DS 3"=w463:bool, "DS 4"=w470:bool, "DS 5"=w469:bool, "DS 6"=w468:bool, "DS 7"=w467:bool, "DS 16"=w466:bool, "DS 17"=w465:bool, "DS 18"=w462:bool, "DS 19"=w461:bool, "DS 20"=w460:bool, "DS 21"=w459:bool)
                                n252 = Compound Arithmetic op=AND(w464, w463, w470, w469, w468, w467, w466, w465, w462, w461, w460, w459) -> (w471:bool)
                              }
                              frame "PHYY5071-2" {
                                n253 = Unbundle By Name(w486) -> ("DS 2"=w478:bool, "DS 3"=w477:bool, "DS 4"=w484:bool, "DS 5"=w483:bool, "DS 6"=w482:bool, "DS 7"=w481:bool, "DS 16"=w480:bool, "DS 17"=w479:bool, "DS 18"=w476:bool, "DS 19"=w475:bool, "DS 20"=w474:bool, "DS 21"=w473:bool)
                                n254 = Compound Arithmetic op=AND(w478, w477, w484, w483, w482, w481, w480, w479, w476, w475, w474, w473) -> (w485:bool)
                              }
                            }
                            n255 = case shown="True" w412 {
                              tunnel: w412 -> [_ _]
                              frame False {
                              }
                              frame True {
                                n256 = Wait (ms)(milliseconds to wait=u32 250) -> ()  [unwired: 1 out]
                              }
                            }
                            "Cluster" <- w413
                          }
                          frame True {
                            n257 = property class="Instr"(reference=w498, error in=w488) -> (reference out=w497:refnum<visa-resource-name>, error out=w496:errorcluster, "Serial Settings:Number of Bytes at Serial Port"=w495:u32)
                            n258 = Not Equal To 0?(x=w495) -> (x != 0?=w494:bool)
                            n259 = case shown="True" w494 {
                              tunnel: w497 -> [w501 w519]
                              tunnel: w495 -> [_ w518]
                              tunnel: w496 -> [w500 w517]
                              tunnel: [w501 w515] -> w493
                              tunnel: [w500 w514] -> w492
                              tunnel: [w499 w502] -> w491
                              tunnel: w490 -> [w499 w503]
                              frame False {
                              }
                              frame True {
                                n260 = VISA Read(VISA resource name=w519, byte count=w518, error in (no error)=w517) -> (VISA resource name out=w515:refnum<visa-resource-name>, read buffer=w516:string, error out=w514:errorcluster)  [unwired: 1 out]
                                n261 = String To Byte Array(string=w516) -> (unsigned byte array=w504:u8[])
                                "Serial In" <- w504
                                n262 = Index Array(array=w504, index #1=u32 0 ("milliseconds to wait"), index #2=1 ("index")) -> (element #1=w513:u8, element #2=w509:u8)
                                n263 = Equal?(x=u8 165 ("index"), y=w513) -> (x = y?=w507:bool)
                                n264 = Equal?(x=w509, y=u8 1 ("index")) -> (x = y?=w506:bool)
                                n265 = And(x=w507, y=w506) -> (x .and. y?=w505:bool)
                                n266 = case shown="True" w505 {
                                tunnel: w504 -> [_ w526]
                                tunnel: w503 -> [w520 w523]
                                tunnel: [w520 w522] -> w502
                                frame False {
                                }
                                frame True {
                                n267 = Index Array(array=w526, index=4) -> (element=w524:u8)
                                n268 = case shown="3" w524 {
                                tunnel: w523 -> [w527 w533 w539 w545 w551 w557 w563 w569 w575 w581 w587 w593 w599 w605 w611 w617 w623 w629 w635 w641 w647 w653]
                                tunnel: [w527 w532 w538 w544 w550 w556 w562 w568 w574 w580 w586 w592 w598 w604 w610 w616 w622 w628 w634 w640 w646 w652] -> w522
                                tunnel: u32 16860 -> [_ w528 w534 w540 w546 w552 w558 w564 w570 w576 w582 w588 w595 w600 w606 w612 w618 w624 w630 w636 w642 w648]
                                frame 0, Default {
                                }
                                frame 1 {
                                n269 = Bundle(w528, w528) -> (w529:cluster{u32, u32})  [unwired: 1 in]
                                n270 = Bundle By Name(cluster=w533, "DS 1"=TRUE) -> (w532:T2)
                                n271 = Build Array(w529) -> (w530:cluster{u32, u32}[])
                                n272 = property on="DS 1" class="Bool (strict)"("Colors [4]"=w530) -> ()  [unwired: 2 in, 2 out]
                                }
                                frame 2 {
                                n273 = Bundle(w534, w534) -> (w535:cluster{u32, u32})  [unwired: 1 in]
                                n274 = Bundle By Name(cluster=w539, "DS 2"=TRUE ("DS 1")) -> (w538:T2)
                                n275 = Build Array(w535) -> (w536:cluster{u32, u32}[])
                                n276 = property on="DS 2" class="Bool (strict)"("Colors [4]"=w536) -> ()  [unwired: 2 in, 2 out]
                                }
                                frame 3 {
                                n277 = Bundle(w540, w540) -> (w541:cluster{u32, u32})  [unwired: 1 in]
                                n278 = Bundle By Name(cluster=w545, "DS 3"=TRUE ("DS 1")) -> (w544:T2)
                                n279 = Build Array(w541) -> (w542:cluster{u32, u32}[])
                                n280 = property on="DS 3" class="Bool (strict)"("Colors [4]"=w542) -> ()  [unwired: 2 in, 2 out]
                                }
                                frame 4 {
                                n281 = Bundle(w546, w546) -> (w547:cluster{u32, u32})  [unwired: 1 in]
                                n282 = Bundle By Name(cluster=w551, "DS 4"=TRUE ("DS 1")) -> (w550:T2)
                                n283 = Build Array(w547) -> (w548:cluster{u32, u32}[])
                                n284 = property on="DS 4" class="Bool (strict)"("Colors [4]"=w548) -> ()  [unwired: 2 in, 2 out]
                                }
                                frame 5 {
                                n285 = Bundle(w552, w552) -> (w553:cluster{u32, u32})  [unwired: 1 in]
                                n286 = Bundle By Name(cluster=w557, "DS 5"=TRUE ("DS 1")) -> (w556:T2)
                                n287 = Build Array(w553) -> (w554:cluster{u32, u32}[])
                                n288 = property on="DS 5" class="Bool (strict)"("Colors [4]"=w554) -> ()  [unwired: 2 in, 2 out]
                                }
                                frame 6 {
                                n289 = Bundle(w558, w558) -> (w559:cluster{u32, u32})  [unwired: 1 in]
                                n290 = Bundle By Name(cluster=w563, "DS 6"=TRUE ("DS 1")) -> (w562:T2)
                                n291 = Build Array(w559) -> (w560:cluster{u32, u32}[])
                                n292 = property on="DS 6" class="Bool (strict)"("Colors [4]"=w560) -> ()  [unwired: 2 in, 2 out]
                                }
                                frame 7 {
                                n293 = Bundle(w564, w564) -> (w565:cluster{u32, u32})  [unwired: 1 in]
                                n294 = Bundle By Name(cluster=w569, "DS 7"=TRUE ("DS 1")) -> (w568:T2)
                                n295 = Build Array(w565) -> (w566:cluster{u32, u32}[])
                                n296 = property on="DS 7" class="Bool (strict)"("Colors [4]"=w566) -> ()  [unwired: 2 in, 2 out]
                                }
                                frame 8 {
                                n297 = Bundle(w570, w570) -> (w571:cluster{u32, u32})  [unwired: 1 in]
                                n298 = Bundle By Name(cluster=w575, "DS 8"=TRUE ("DS 1")) -> (w574:T2)
                                n299 = Build Array(w571) -> (w572:cluster{u32, u32}[])
                                n300 = property on="DS 8" class="Bool (strict)"("Colors [4]"=w572) -> ()  [unwired: 2 in, 2 out]
                                }
                                frame 9 {
                                n301 = Bundle(w576, w576) -> (w577:cluster{u32, u32})  [unwired: 1 in]
                                n302 = Bundle By Name(cluster=w581, "DS 9"=TRUE ("DS 1")) -> (w580:T2)
                                n303 = Build Array(w577) -> (w578:cluster{u32, u32}[])
                                n304 = property on="DS 9" class="Bool (strict)"("Colors [4]"=w578) -> ()  [unwired: 2 in, 2 out]
                                }
                                frame 10 {
                                n305 = Bundle(w582, w582) -> (w583:cluster{u32, u32})  [unwired: 1 in]
                                n306 = Bundle By Name(cluster=w587, "DS 10"=TRUE ("DS 1")) -> (w586:T2)
                                n307 = Build Array(w583) -> (w584:cluster{u32, u32}[])
                                n308 = property on="DS 10" class="Bool (strict)"("Colors [4]"=w584) -> ()  [unwired: 2 in, 2 out]
                                }
                                frame 11 {
                                n309 = Bundle(w588, w588) -> (w589:cluster{u32, u32})  [unwired: 1 in]
                                n310 = Bundle By Name(cluster=w593, "DS 11"=TRUE ("DS 1")) -> (w592:T2)
                                n311 = Build Array(w589) -> (w590:cluster{u32, u32}[])
                                n312 = property on="DS 11" class="Bool (strict)"("Colors [4]"=w590) -> ()  [unwired: 2 in, 2 out]
                                }
                                frame 12 {
                                n313 = Bundle(w595, w595) -> (w596:cluster{u32, u32})  [unwired: 1 in]
                                n314 = Bundle By Name(cluster=w599, "DS 12"=TRUE ("DS 1")) -> (w598:T2)
                                n315 = Build Array(w596) -> (w594:cluster{u32, u32}[])
                                n316 = property on="DS 12" class="Bool (strict)"("Colors [4]"=w594) -> ()  [unwired: 2 in, 2 out]
                                }
                                frame 13 {
                                n317 = Bundle(w600, w600) -> (w601:cluster{u32, u32})  [unwired: 1 in]
                                n318 = Bundle By Name(cluster=w605, "DS 13"=TRUE ("DS 1")) -> (w604:T2)
                                n319 = Build Array(w601) -> (w602:cluster{u32, u32}[])
                                n320 = property on="DS 13" class="Bool (strict)"("Colors [4]"=w602) -> ()  [unwired: 2 in, 2 out]
                                }
                                frame 14 {
                                n321 = Bundle(w606, w606) -> (w607:cluster{u32, u32})  [unwired: 1 in]
                                n322 = Bundle By Name(cluster=w611, "DS 14"=TRUE ("DS 1")) -> (w610:T2)
                                n323 = Build Array(w607) -> (w608:cluster{u32, u32}[])
                                n324 = property on="DS 14" class="Bool (strict)"("Colors [4]"=w608) -> ()  [unwired: 2 in, 2 out]
                                }
                                frame 15 {
                                n325 = Bundle(w612, w612) -> (w613:cluster{u32, u32})  [unwired: 1 in]
                                n326 = Bundle By Name(cluster=w617, "DS 15"=TRUE ("DS 1")) -> (w616:T2)
                                n327 = Build Array(w613) -> (w614:cluster{u32, u32}[])
                                n328 = property on="DS 15" class="Bool (strict)"("Colors [4]"=w614) -> ()  [unwired: 2 in, 2 out]
                                }
                                frame 16 {
                                n329 = Bundle(w618, w618) -> (w619:cluster{u32, u32})  [unwired: 1 in]
                                n330 = Build Array(w619) -> (w620:cluster{u32, u32}[])
                                n331 = Bundle By Name(cluster=w623, "DS 16"=TRUE ("DS 1")) -> (w622:T2)
                                n332 = property on="DS 16" class="Bool (strict)"("Colors [4]"=w620) -> ()  [unwired: 2 in, 2 out]
                                }
                                frame 17 {
                                n333 = Bundle(w624, w624) -> (w625:cluster{u32, u32})  [unwired: 1 in]
                                n334 = Bundle By Name(cluster=w629, "DS 17"=TRUE ("DS 1")) -> (w628:T2)
                                n335 = Build Array(w625) -> (w626:cluster{u32, u32}[])
                                n336 = property on="DS 17" class="Bool (strict)"("Colors [4]"=w626) -> ()  [unwired: 2 in, 2 out]
                                }
                                frame 18 {
                                n337 = Bundle(w630, w630) -> (w631:cluster{u32, u32})  [unwired: 1 in]
                                n338 = Bundle By Name(cluster=w635, "DS 18"=TRUE ("DS 1")) -> (w634:T2)
                                n339 = Build Array(w631) -> (w632:cluster{u32, u32}[])
                                n340 = property on="DS 18" class="Bool (strict)"("Colors [4]"=w632) -> ()  [unwired: 2 in, 2 out]
                                }
                                frame 19 {
                                n341 = Bundle(w636, w636) -> (w637:cluster{u32, u32})  [unwired: 1 in]
                                n342 = Build Array(w637) -> (w638:cluster{u32, u32}[])
                                n343 = Bundle By Name(cluster=w641, "DS 19"=TRUE ("DS 1")) -> (w640:T2)
                                n344 = property on="DS 19" class="Bool (strict)"("Colors [4]"=w638) -> ()  [unwired: 2 in, 2 out]
                                }
                                frame 20 {
                                n345 = Bundle(w642, w642) -> (w643:cluster{u32, u32})  [unwired: 1 in]
                                n346 = Bundle By Name(cluster=w647, "DS 20"=TRUE ("DS 1")) -> (w646:T2)
                                n347 = Build Array(w643) -> (w644:cluster{u32, u32}[])
                                n348 = property on="DS 20" class="Bool (strict)"("Colors [4]"=w644) -> ()  [unwired: 2 in, 2 out]
                                }
                                frame 21 {
                                n349 = Bundle(w648, w648) -> (w649:cluster{u32, u32})  [unwired: 1 in]
                                n350 = Bundle By Name(cluster=w653, "DS 21"=TRUE ("DS 1")) -> (w652:T2)
                                n351 = Build Array(w649) -> (w650:cluster{u32, u32}[])
                                n352 = property on="DS 21" class="Bool (strict)"("Colors [4]"=w650) -> ()  [unwired: 2 in, 2 out]
                                }
                                }
                                }
                                }
                              }
                            }
                          }
                        }
                        n353 = Less Than 0?(x=w392) -> (x < 0?=w391:bool)
                        n354 = Compound Arithmetic op=OR(w388, "btnStop", w391) -> (w395:bool)
                        n355 = case shown="True" "btnStop" {
                          tunnel: [T5."LED TEST" T5."DISABLE POWER"] -> w389
                          frame False {
                          }
                          frame True {
                          }
                        }
                      }
                      n356 = case shown="True" w372 {
                        tunnel: [TRUE ("bKeys") _] -> w371
                        frame False {
                        }
                        frame True {
                        }
                      }
                      "bKeys" <- w371
                    }
                    frame "LED TEST" {
                      n357 = property on="String" class="Str"(error in=w658, "Value"="LED test..." ("String")) -> (error out=w657:errorcluster)  [unwired: 1 in, 1 out]
                      n358 = for {
                        N: 2 -> [_]
                        tunnel: w663 -> [w683]
                        tunnel: w669 -> [w676]
                        tunnel: w657 -> [w675]
                        tunnel: [w682] -> w668
                        tunnel: [w681] -> w667
                        tunnel: [w679] -> w666
                        shift-right: [w677] -> _
                        shift-left: TRUE ("Enable") -> [w678]
                        tunnel: [w672] -> _
                        tunnel: w662 -> [w673]
                        tunnel: [w672] -> w655
                        tunnel: w654 -> [w671]
                        i -> [w674]
                        n359 = case shown="0, Default" w674 {
                          tunnel: [w693 _] -> w684
                          tunnel: [w692 w920] -> w682
                          tunnel: [w691 w919] -> w680
                          tunnel: w678 -> [w690 _]
                          tunnel: w676 -> [w689 w922]
                          tunnel: w675 -> [w688 w921]
                          tunnel: w673 -> [w687 w923]
                          tunnel: [_ w918] -> w672
                          tunnel: w671 -> [w685 _]
                          frame 0, Default {
                            # "Turn on the LED's according to the part."
                            n360 = case shown="\"PHYY5037-1\"" w685 {
                              tunnel: [w702 w747 w792 w837 w882] -> w693
                              tunnel: [w701 w746 w791 w836 w881] -> w692
                              tunnel: [w700 w745 w790 w835 w880] -> w691
                              tunnel: w690 -> [w699 w744 w789 w834 w879]
                              tunnel: w689 -> [w698 w743 w788 w833 w878]
                              tunnel: w688 -> [w697 w742 w787 w832 w877]
                              tunnel: w687 -> [w695 w740 w785 w830 w875]
                              tunnel: [w694 w739 w784 w829 w874] -> w686
                              frame "PHYY5042-1", Default {
                                n361 = for {
                                N: 10 -> [_]
                                tunnel: [w725] -> w702
                                tunnel: [w718] -> w701
                                tunnel: [w706] -> w700
                                tunnel: w699 -> [w717]
                                tunnel: w698 -> [w716]
                                tunnel: w697 -> [w715]
                                tunnel: w695 -> [w705]
                                tunnel: [w704] -> w694 mode=indexing
                                i -> [w714]
                                n362 = Increment(x=w714) -> (x+1=w713:i32)
                                n363 = Wait (ms)(milliseconds to wait=u32 15) -> ()  [unwired: 1 out]
                                n364 = case shown="\"LED_CMD\"" enum16{"KYPD_CMD", "LED_CMD", "KEY_ERROR_CMD"}."LED_CMD" ("CMD") {
                                tunnel: [1 2 3] -> w724
                                tunnel: [w732 w734 FALSE ("Enable")] -> w725
                                tunnel: w717 -> [w732 w734 _]
                                frame "KYPD_CMD", Default {
                                }
                                frame "LED_CMD" {
                                }
                                frame "KEY_ERROR_CMD" {
                                }
                                }
                                n365 = Add(x=w724, y=w713) -> (x+y=w720:i32)
                                n366 = Build Array(u8 165, u8 4, w724, w713, w720) -> (w703:i32[])
                                n367 = Byte Array To String(unsigned byte array=w703) -> (string=w719:string)
                                n368 = property on="Serial Out" class="Arr (strict)"("Value"=w703) -> ()  [unwired: 2 in, 2 out]
                                n369 = VISA Write(VISA resource name=w716, write buffer=w719, error in (no error)=w715) -> (VISA resource name out=w718:refnum<visa-resource-name>, error out=w707:errorcluster)  [unwired: 1 out]
                                n370 = for {
                                N: 2 -> [w728]
                                tunnel: w707 -> [w731]
                                tunnel: [w729] -> w710 mode=indexing
                                tunnel: [w728] -> w708
                                tunnel: [w727] -> w706
                                tunnel: w705 -> [w726]
                                n371 = call <instrlib>:"Measure.vi"("error in (no error)"=w731, "Measurement Type (Voltage)"="MEAS:CURR?", "VISA resource name"=w726) -> ("error out"=w727:errorcluster, "Measurement"=w729:dbl)  [unwired: 6 in, 1 out]
                                }
                                n372 = Add Array Elements(numeric array=w710) -> (sum=w709:dbl)
                                n373 = Divide(x=w709, y=w708) -> (x/y=w704:dbl)
                                }
                              }
                              frame "PHYY5037-1" {
                                n374 = for {
                                N: 6 -> [_]
                                tunnel: [w770] -> w747
                                tunnel: [w763] -> w746
                                tunnel: [w753] -> w745
                                tunnel: w744 -> [w762]
                                tunnel: w743 -> [w761]
                                tunnel: w742 -> [w760]
                                tunnel: w740 -> [w752]
                                tunnel: [w751] -> w739 mode=indexing
                                shift-right: [w748] -> _
                                shift-left: 2 -> [w749]
                                n375 = Wait (ms)(milliseconds to wait=u32 15) -> ()  [unwired: 1 out]
                                n376 = case shown="\"LED_CMD\"" enum16{"KYPD_CMD", "LED_CMD", "KEY_ERROR_CMD"}."LED_CMD" ("CMD") {
                                tunnel: [1 2 3] -> w769
                                tunnel: [w777 w779 FALSE ("Enable")] -> w770
                                tunnel: w762 -> [w777 w779 _]
                                frame "KYPD_CMD", Default {
                                }
                                frame "LED_CMD" {
                                }
                                frame "KEY_ERROR_CMD" {
                                }
                                }
                                n377 = Increment(x=w749) -> (x+1=w748:i32)
                                n378 = Add(x=w769, y=w749) -> (x+y=w765:i32)
                                n379 = Build Array(u8 165, u8 4, w769, w749, w765) -> (w750:i32[])
                                n380 = Byte Array To String(unsigned byte array=w750) -> (string=w764:string)
                                n381 = property on="Serial Out" class="Arr (strict)"("Value"=w750) -> ()  [unwired: 2 in, 2 out]
                                n382 = VISA Write(VISA resource name=w761, write buffer=w764, error in (no error)=w760) -> (VISA resource name out=w763:refnum<visa-resource-name>, error out=w754:errorcluster)  [unwired: 1 out]
                                n383 = for {
                                N: 2 -> [w773]
                                tunnel: w754 -> [w776]
                                tunnel: [w774] -> w757 mode=indexing
                                tunnel: [w773] -> w755
                                tunnel: [w772] -> w753
                                tunnel: w752 -> [w771]
                                n384 = call <instrlib>:"Measure.vi"("error in (no error)"=w776, "Measurement Type (Voltage)"="MEAS:CURR?", "VISA resource name"=w771) -> ("error out"=w772:errorcluster, "Measurement"=w774:dbl)  [unwired: 6 in, 1 out]
                                }
                                n385 = Add Array Elements(numeric array=w757) -> (sum=w756:dbl)
                                n386 = Divide(x=w756, y=w755) -> (x/y=w751:dbl)
                                }
                              }
                              frame "PHYY5110-1" {
                                n387 = for {
                                N: 6 -> [_]
                                tunnel: [w815] -> w792
                                tunnel: [w808] -> w791
                                tunnel: [w798] -> w790
                                tunnel: w789 -> [w807]
                                tunnel: w788 -> [w806]
                                tunnel: w787 -> [w805]
                                tunnel: w785 -> [w797]
                                tunnel: [w796] -> w784 mode=indexing
                                shift-right: [w793] -> _
                                shift-left: 2 -> [w794]
                                n388 = Wait (ms)(milliseconds to wait=u32 15) -> ()  [unwired: 1 out]
                                n389 = case shown="\"LED_CMD\"" enum16{"KYPD_CMD", "LED_CMD", "KEY_ERROR_CMD"}."LED_CMD" ("CMD") {
                                tunnel: [1 2 3] -> w814
                                tunnel: [w822 w824 FALSE ("Enable")] -> w815
                                tunnel: w807 -> [w822 w824 _]
                                frame "KYPD_CMD", Default {
                                }
                                frame "LED_CMD" {
                                }
                                frame "KEY_ERROR_CMD" {
                                }
                                }
                                n390 = Increment(x=w794) -> (x+1=w793:i32)
                                n391 = Add(x=w814, y=w794) -> (x+y=w810:i32)
                                n392 = Build Array(u8 165, u8 4, w814, w794, w810) -> (w795:i32[])
                                n393 = Byte Array To String(unsigned byte array=w795) -> (string=w809:string)
                                n394 = property on="Serial Out" class="Arr (strict)"("Value"=w795) -> ()  [unwired: 2 in, 2 out]
                                n395 = VISA Write(VISA resource name=w806, write buffer=w809, error in (no error)=w805) -> (VISA resource name out=w808:refnum<visa-resource-name>, error out=w799:errorcluster)  [unwired: 1 out]
                                n396 = for {
                                N: 2 -> [w818]
                                tunnel: w799 -> [w821]
                                tunnel: [w819] -> w802 mode=indexing
                                tunnel: [w818] -> w800
                                tunnel: [w817] -> w798
                                tunnel: w797 -> [w816]
                                n397 = call <instrlib>:"Measure.vi"("error in (no error)"=w821, "Measurement Type (Voltage)"="MEAS:CURR?", "VISA resource name"=w816) -> ("error out"=w817:errorcluster, "Measurement"=w819:dbl)  [unwired: 6 in, 1 out]
                                }
                                n398 = Add Array Elements(numeric array=w802) -> (sum=w801:dbl)
                                n399 = Divide(x=w801, y=w800) -> (x/y=w796:dbl)
                                }
                              }
                              frame "PHYY5110-2" {
                                n400 = for {
                                N: 6 -> [_]
                                tunnel: [w860] -> w837
                                tunnel: [w853] -> w836
                                tunnel: [w843] -> w835
                                tunnel: w834 -> [w852]
                                tunnel: w833 -> [w851]
                                tunnel: w832 -> [w850]
                                tunnel: w830 -> [w842]
                                tunnel: [w841] -> w829 mode=indexing
                                shift-right: [w838] -> _
                                shift-left: 2 -> [w839]
                                n401 = Wait (ms)(milliseconds to wait=u32 15) -> ()  [unwired: 1 out]
                                n402 = case shown="\"LED_CMD\"" enum16{"KYPD_CMD", "LED_CMD", "KEY_ERROR_CMD"}."LED_CMD" ("CMD") {
                                tunnel: [1 2 3] -> w859
                                tunnel: [w867 w869 FALSE ("Enable")] -> w860
                                tunnel: w852 -> [w867 w869 _]
                                frame "KYPD_CMD", Default {
                                }
                                frame "LED_CMD" {
                                }
                                frame "KEY_ERROR_CMD" {
                                }
                                }
                                n403 = Increment(x=w839) -> (x+1=w838:i32)
                                n404 = Add(x=w859, y=w839) -> (x+y=w855:i32)
                                n405 = Build Array(u8 165, u8 4, w859, w839, w855) -> (w840:i32[])
                                n406 = Byte Array To String(unsigned byte array=w840) -> (string=w854:string)
                                n407 = property on="Serial Out" class="Arr (strict)"("Value"=w840) -> ()  [unwired: 2 in, 2 out]
                                n408 = VISA Write(VISA resource name=w851, write buffer=w854, error in (no error)=w850) -> (VISA resource name out=w853:refnum<visa-resource-name>, error out=w844:errorcluster)  [unwired: 1 out]
                                n409 = for {
                                N: 2 -> [w863]
                                tunnel: w844 -> [w866]
                                tunnel: [w864] -> w847 mode=indexing
                                tunnel: [w863] -> w845
                                tunnel: [w862] -> w843
                                tunnel: w842 -> [w861]
                                n410 = call <instrlib>:"Measure.vi"("error in (no error)"=w866, "Measurement Type (Voltage)"="MEAS:CURR?", "VISA resource name"=w861) -> ("error out"=w862:errorcluster, "Measurement"=w864:dbl)  [unwired: 6 in, 1 out]
                                }
                                n411 = Add Array Elements(numeric array=w847) -> (sum=w846:dbl)
                                n412 = Divide(x=w846, y=w845) -> (x/y=w841:dbl)
                                }
                              }
                              frame "PHYY5037-2" {
                                n413 = for {
                                N: 6 -> [_]
                                tunnel: [w905] -> w882
                                tunnel: [w898] -> w881
                                tunnel: [w888] -> w880
                                tunnel: w879 -> [w897]
                                tunnel: w878 -> [w896]
                                tunnel: w877 -> [w895]
                                tunnel: w875 -> [w887]
                                tunnel: [w886] -> w874 mode=indexing
                                shift-right: [w883] -> _
                                shift-left: 2 -> [w884]
                                n414 = Wait (ms)(milliseconds to wait=u32 15) -> ()  [unwired: 1 out]
                                n415 = case shown="\"LED_CMD\"" enum16{"KYPD_CMD", "LED_CMD", "KEY_ERROR_CMD"}."LED_CMD" ("CMD") {
                                tunnel: [1 2 3] -> w904
                                tunnel: [w912 w914 FALSE ("Enable")] -> w905
                                tunnel: w897 -> [w912 w914 _]
                                frame "KYPD_CMD", Default {
                                }
                                frame "LED_CMD" {
                                }
                                frame "KEY_ERROR_CMD" {
                                }
                                }
                                n416 = Increment(x=w884) -> (x+1=w883:i32)
                                n417 = Add(x=w904, y=w884) -> (x+y=w900:i32)
                                n418 = Build Array(u8 165, u8 4, w904, w884, w900) -> (w885:i32[])
                                n419 = Byte Array To String(unsigned byte array=w885) -> (string=w899:string)
                                n420 = property on="Serial Out" class="Arr (strict)"("Value"=w885) -> ()  [unwired: 2 in, 2 out]
                                n421 = VISA Write(VISA resource name=w896, write buffer=w899, error in (no error)=w895) -> (VISA resource name out=w898:refnum<visa-resource-name>, error out=w889:errorcluster)  [unwired: 1 out]
                                n422 = for {
                                N: 2 -> [w908]
                                tunnel: w889 -> [w911]
                                tunnel: [w909] -> w892 mode=indexing
                                tunnel: [w908] -> w890
                                tunnel: [w907] -> w888
                                tunnel: w887 -> [w906]
                                n423 = call <instrlib>:"Measure.vi"("error in (no error)"=w911, "Measurement Type (Voltage)"="MEAS:CURR?", "VISA resource name"=w906) -> ("error out"=w907:errorcluster, "Measurement"=w909:dbl)  [unwired: 6 in, 1 out]
                                }
                                n424 = Add Array Elements(numeric array=w892) -> (sum=w891:dbl)
                                n425 = Divide(x=w891, y=w890) -> (x/y=w886:dbl)
                                }
                              }
                            }
                            "dlbLED" <- w686
                          }
                          frame 1 {
                            n426 = stacked-sequence {
                              tunnel: w922 -> [_ _ w940]
                              tunnel: [_ _ w941] -> w920
                              tunnel: w921 -> [w930 _ w943]
                              tunnel: [_ _ w942] -> w919
                              tunnel: [_ w936 _] -> w918
                              tunnel: w923 -> [w924 _ _]
                              frame #0 {
                                n427 = for {
                                N: 10 -> [w931]
                                tunnel: w930 -> [w935]
                                tunnel: w924 -> [w934]
                                tunnel: [w932] -> w928 mode=indexing
                                tunnel: [w931] -> w926
                                n428 = call <instrlib>:"Measure.vi"("error in (no error)"=w935, "Measurement Type (Voltage)"="MEAS:CURR?", "VISA resource name"=w934) -> ("Measurement"=w932:dbl)  [unwired: 6 in, 2 out]
                                }
                                n429 = Add Array Elements(numeric array=w928) -> (sum=w927:dbl)
                                n430 = Divide(x=w927, y=w926) -> (x/y=→"dlbAllLEDs":dbl)
                              }
                              frame #1 {
                                n431 = Two Button Dialog(message="VERIFY ALL LEDS ARE ON.", 1:"NO" ("F button name (\"Cancel\")"), 2:"YES" ("T button name (\"OK\")")) -> (T button?=w936:bool)
                              }
                              frame #2 {
                                w951 = 0
                                # "Turns off all LED's."
                                n432 = case shown="\"LED_CMD\"" enum16{"KYPD_CMD", "LED_CMD", "KEY_ERROR_CMD"}."LED_CMD" ("CMD") {
                                tunnel: [1 2 3] -> w944
                                frame "KYPD_CMD", Default {
                                }
                                frame "LED_CMD" {
                                }
                                frame "KEY_ERROR_CMD" {
                                (unwired) FALSE ("Enable")
                                }
                                }
                                n433 = Add(x=w944, y=w951) -> (x+y=w949:i32)
                                n434 = Build Array(u8 165, u8 4, w944, w951, w949) -> (w946:i32[])
                                "Serial Out 2" <- w946
                                n435 = Byte Array To String(unsigned byte array=w946) -> (string=w950:string)
                                n436 = VISA Write(VISA resource name=w940, write buffer=w950, error in (no error)=w943) -> (VISA resource name out=w941:refnum<visa-resource-name>, error out=w942:errorcluster)  [unwired: 1 out]
                              }
                            }
                          }
                        }
                        n437 = Not(x=w678) -> (.not. x?=w677:bool)
                        n438 = Bundle By Name(cluster=w683, "bLed 0"=w684, "bLed 1"=w684, "bLed 2"=w684, "bLed 3"=w684, "bLed 4"=w684, "bLed 5"=w684, "bLed 6"=w684, "bLed 7"=w684, "bLed 8"=w684, "bLed 9"=w684) -> (w681:T2)
                        n439 = property on="Cluster" class="Clust (strict)"(error in=w680, "Value"=w681) -> (error out=w679:errorcluster)  [unwired: 1 in, 1 out]
                      }
                      n440 = case shown="False" w655 {
                        tunnel: [TRUE _] -> w656
                        frame False {
                        }
                        frame True {
                        }
                      }
                      "bLEDs" <- w656
                    }
                    frame "DISABLE POWER" {
                      n441 = property on="String" class="Str"(error in=w956, "Value"="Disable power..." ("String")) -> (error out=w955:errorcluster)  [unwired: 1 in, 1 out]
                      n442 = call <instrlib>:"Configure Output Enabled.vi"("error in (no error)"=w955, "Output Enabled (F: Off)"=FALSE, "VISA resource name"=w962) -> ("error out"=w960:errorcluster, "VISA resource name out"=w959:refnum<visa-resource-name>)  [unwired: 7 in]
                    }
                    frame "TEST END" {
                      n443 = property on="enumPart" class="Enum (strict)"() -> ("RingText.Text"=w964:string)  [unwired: 2 in, 2 out]
                      n444 = property on="String" class="Str"(error in=w979, "Value"="Log data..." ("String")) -> (error out=w978:errorcluster)  [unwired: 1 in, 1 out]
                      n445 = property on="dlbLED" class="Arr (strict)"(error in=w978) -> (error out=w992:errorcluster, "Value"=w965:dbl[])  [unwired: 1 in, 1 out]
                      n446 = property on="dlbAllLEDs" class="DigNum (strict)"(error in=w992) -> (error out=w985:errorcluster, "Value"=w989:dbl)  [unwired: 1 in, 1 out]
                      n447 = Array Size(array=w965) -> (size(s)=w968:i32)
                      n448 = Equal To 0?(x=w968) -> (x = 0?=w967:bool)
                      n449 = property on="Employee ID" class="Str"(error in=w985) -> (error out=w983:errorcluster, "Value"=w984:string)  [unwired: 1 in, 1 out]
                      n450 = case shown="True" w967 {
                        tunnel: [w1006 w1007] -> w966
                        tunnel: w965 -> [w1006 w1008]
                        frame False {
                        }
                        frame True {
                          n451 = Reshape Array(w1008, 10 ("dimension size")) -> (w1007:dbl[])
                        }
                      }
                      n452 = property on="SW VER" class="Str"(error in=w983) -> (error out=w974:errorcluster, "Value"=w982:string)  [unwired: 1 in, 1 out]
                      n453 = property on="bDomeClosed" class="Bool (strict)"(error in=w974) -> (error out=w973:errorcluster, "Value"=w972:bool)  [unwired: 1 in, 1 out]
                      n454 = Not(x=w972) -> (.not. x?=w971:bool)
                      n455 = property on="bKeys" class="Bool (strict)"(error in=w973) -> (error out=w1002:errorcluster, "Value"=w987:bool)  [unwired: 1 in, 1 out]
                      n456 = Not(x=w987) -> (.not. x?=w970:bool)
                      n457 = property on="bLEDs" class="Bool (strict)"(error in=w1002) -> (error out=w1001:errorcluster, "Value"=w986:bool)  [unwired: 1 in, 1 out]
                      n458 = Not(x=w986) -> (.not. x?=w969:bool)
                      n459 = Compound Arithmetic op=AND(w969, w970, w971) -> (w988:bool)
                      n460 = case shown="False" w988 {
                        tunnel: [2 1] -> w993
                        frame False {
                        }
                        frame True {
                        }
                      }
                      n461 = Bundle By Name(cluster=T6 {"dlbLED"=[], "dlbAllLEDs"=0.0, "Pass/Fail"=FALSE, "Keys"=FALSE, "LEDS"=FALSE, "Employee ID"="", "Part Number"="", "SW Version"=""} ("Cluster"), "dlbLED"=w966, "dlbAllLEDs"=w989, "Pass/Fail"=w988, "Keys"=w987, "LEDS"=w986, "Employee ID"=w984, "Part Number"=w964, "SW Version"=w982) -> (w991:T6)
                      n462 = call "Write Data To Table.vi"("Cluster"=w991, "file path (dialog if empty)"=w981) -> ()  [unwired: 2 in]
                      n463 = Index Array(array=u32[] [13816530, 1244928, 16711680], index=w993) -> (element=w996:u32)
                      n464 = Bundle(w996, w996) -> (w995:cluster{u32, u32})  [unwired: 1 in]
                      n465 = Build Array(w995) -> (w994:cluster{u32, u32}[])
                      n466 = Select(t="PASS" ("Boolean Text.Text"), s=w988, f="FAIL" ("Boolean Text.Text")) -> (s? t:f=w999:string)
                      n467 = property on="bPassFail" class="Bool (strict)"(error in=w1001, "Value"=w988, "BoolText.Text"=w999, "Colors [4]"=w994) -> (error out=w976:errorcluster)  [unwired: 1 in, 1 out]
                      n468 = property on="String" class="Str"(error in=w976, "Value"="" ("String")) -> (error out=w975:errorcluster)  [unwired: 1 in, 1 out]
                    }
                  }
                }
                n469 = VISA Close(VISA resource name=w226, error in (no error)=w225) -> (error out=w220:errorcluster)
                n470 = call <instrlib>:"Close.vi"("error in (no error)"=w220, "VISA resource name"=w218) -> ("error out"=w219:errorcluster)  [unwired: 9 in]
              }
              frame Error {
                n471 = Unbundle By Name(w1021) -> ("source"=w1020:string)
                n472 = property on="Boolean" class="Bool (strict)"("Visible"=TRUE) -> (error out=w1017:errorcluster)  [unwired: 2 in, 1 out]
                n473 = property on="Boolean" class="Bool (strict)"(error in=w1017, "Blinking"=TRUE) -> (error out=w1016:errorcluster)  [unwired: 1 in, 1 out]
                n474 = Concatenate Strings("ERROR: " ("string"), w1020) -> (w1019:string)
                n475 = stacked-sequence {
                  tunnel: w1019 -> [w1025 _]
                  tunnel: w1016 -> [_ w1026]
                  tunnel: [_ w1026] -> w1013
                  tunnel: [w1023 _] -> w1012
                  frame #0 {
                    n476 = One Button Dialog(message=w1025) -> (true=w1024:bool)  [unwired: 1 in]
                    n477 = Not(x=w1024) -> (.not. x?=w1023:bool)
                  }
                  frame #1 {
                  }
                }
                n478 = property on="Boolean" class="Bool (strict)"(error in=w1013, "Visible"=w1012) -> (error out=w1014:errorcluster)  [unwired: 1 in, 1 out]
                n479 = property on="Boolean" class="Bool (strict)"(error in=w1014, "Blinking"=w1012) -> ()  [unwired: 1 in, 2 out]
              }
            }
          }
          frame Error {
            n480 = Unbundle By Name(w1027) -> ("source"=w1029:string)
            n481 = Concatenate Strings("ERROR: " ("string"), w1029) -> (w1028:string)
            n482 = One Button Dialog(message=w1028) -> ()  [unwired: 1 in, 1 out]
          }
        }
        n483 = call <vilib>:"Clear Errors.vi"("error in (no error)"=w200) -> ("error out"=w199:errorcluster)  [unwired: 6 in]
        n484 = property on="btnStart" class="Bool (strict)"(error in=w199, "DisabledEnum"=T3."Enabled" ("Disabled"), "Value"=w197) -> (error out=w198:errorcluster)  [unwired: 1 in, 1 out]
        n485 = property on="btnStop" class="Bool (strict)"(error in=w198, "Value"=w197) -> (error out=w196:errorcluster)  [unwired: 1 in, 1 out]
      }
    }
    "SW VER" <- "C" ("SW VER")
  }
  n486 = disable-structure shown="Disabled" {
    frame Disabled {
      n487 = for {
        N: 21 -> [_]
        tunnel: u32 7447295 -> [w1035]
        tunnel: [w1034] -> _
        tunnel: _ -> [w1033]
        i -> [w1036]
        n488 = case shown="2" w1036 {
          tunnel: w1035 -> [w1037 w1040 w1043 w1046 w1049 w1052 w1055 w1058 w1061 w1064 w1067 w1070 w1073 w1076 w1079 w1082 w1085 w1088 w1091 w1094 w1098]
          tunnel: [_ _ _ _ _ _ _ _ _ _ _ _ _ _ _ _ _ _ _ _ w1097] -> w1034
          tunnel: w1033 -> [_ _ _ _ _ _ _ _ _ _ _ _ _ _ _ _ _ _ _ _ _]
          frame 0, Default {
            n489 = Bundle(w1037, w1037) -> (w1039:cluster{u32, u32})  [unwired: 1 in]
            n490 = Build Array(w1039) -> (w1038:cluster{u32, u32}[])
            n491 = property on="DS 1" class="Bool (strict)"("Colors [4]"=w1038) -> ()  [unwired: 2 in, 2 out]
          }
          frame 1 {
            n492 = Bundle(w1040, w1040) -> (w1042:cluster{u32, u32})  [unwired: 1 in]
            n493 = Build Array(w1042) -> (w1041:cluster{u32, u32}[])
            n494 = property on="DS 2" class="Bool (strict)"("Colors [4]"=w1041) -> ()  [unwired: 2 in, 2 out]
          }
          frame 2 {
            n495 = Bundle(w1043, w1043) -> (w1045:cluster{u32, u32})  [unwired: 1 in]
            n496 = Build Array(w1045) -> (w1044:cluster{u32, u32}[])
            n497 = property on="DS 3" class="Bool (strict)"("Colors [4]"=w1044) -> ()  [unwired: 2 in, 2 out]
          }
          frame 3 {
            n498 = Bundle(w1046, w1046) -> (w1047:cluster{u32, u32})  [unwired: 1 in]
            n499 = Build Array(w1047) -> (w1048:cluster{u32, u32}[])
            n500 = property on="DS 4" class="Bool (strict)"("Colors [4]"=w1048) -> ()  [unwired: 2 in, 2 out]
          }
          frame 4 {
            n501 = Bundle(w1049, w1049) -> (w1051:cluster{u32, u32})  [unwired: 1 in]
            n502 = Build Array(w1051) -> (w1050:cluster{u32, u32}[])
            n503 = property on="DS 5" class="Bool (strict)"("Colors [4]"=w1050) -> ()  [unwired: 2 in, 2 out]
          }
          frame 5 {
            n504 = Bundle(w1052, w1052) -> (w1054:cluster{u32, u32})  [unwired: 1 in]
            n505 = Build Array(w1054) -> (w1053:cluster{u32, u32}[])
            n506 = property on="DS 6" class="Bool (strict)"("Colors [4]"=w1053) -> ()  [unwired: 2 in, 2 out]
          }
          frame 6 {
            n507 = Bundle(w1055, w1055) -> (w1057:cluster{u32, u32})  [unwired: 1 in]
            n508 = Build Array(w1057) -> (w1056:cluster{u32, u32}[])
            n509 = property on="DS 7" class="Bool (strict)"("Colors [4]"=w1056) -> ()  [unwired: 2 in, 2 out]
          }
          frame 7 {
            n510 = Bundle(w1058, w1058) -> (w1060:cluster{u32, u32})  [unwired: 1 in]
            n511 = Build Array(w1060) -> (w1059:cluster{u32, u32}[])
            n512 = property on="DS 8" class="Bool (strict)"("Colors [4]"=w1059) -> ()  [unwired: 2 in, 2 out]
          }
          frame 8 {
            n513 = Bundle(w1061, w1061) -> (w1063:cluster{u32, u32})  [unwired: 1 in]
            n514 = Build Array(w1063) -> (w1062:cluster{u32, u32}[])
            n515 = property on="DS 9" class="Bool (strict)"("Colors [4]"=w1062) -> ()  [unwired: 2 in, 2 out]
          }
          frame 9 {
            n516 = Bundle(w1064, w1064) -> (w1066:cluster{u32, u32})  [unwired: 1 in]
            n517 = Build Array(w1066) -> (w1065:cluster{u32, u32}[])
            n518 = property on="DS 10" class="Bool (strict)"("Colors [4]"=w1065) -> ()  [unwired: 2 in, 2 out]
          }
          frame 10 {
            n519 = Bundle(w1067, w1067) -> (w1069:cluster{u32, u32})  [unwired: 1 in]
            n520 = Build Array(w1069) -> (w1068:cluster{u32, u32}[])
            n521 = property on="DS 11" class="Bool (strict)"("Colors [4]"=w1068) -> ()  [unwired: 2 in, 2 out]
          }
          frame 11 {
            n522 = Bundle(w1070, w1070) -> (w1071:cluster{u32, u32})  [unwired: 1 in]
            n523 = Build Array(w1071) -> (w1072:cluster{u32, u32}[])
            n524 = property on="DS 12" class="Bool (strict)"("Colors [4]"=w1072) -> ()  [unwired: 2 in, 2 out]
          }
          frame 12 {
            n525 = Bundle(w1073, w1073) -> (w1075:cluster{u32, u32})  [unwired: 1 in]
            n526 = Build Array(w1075) -> (w1074:cluster{u32, u32}[])
            n527 = property on="DS 13" class="Bool (strict)"("Colors [4]"=w1074) -> ()  [unwired: 2 in, 2 out]
          }
          frame 13 {
            n528 = Bundle(w1076, w1076) -> (w1078:cluster{u32, u32})  [unwired: 1 in]
            n529 = Build Array(w1078) -> (w1077:cluster{u32, u32}[])
            n530 = property on="DS 14" class="Bool (strict)"("Colors [4]"=w1077) -> ()  [unwired: 2 in, 2 out]
          }
          frame 14 {
            n531 = Bundle(w1079, w1079) -> (w1081:cluster{u32, u32})  [unwired: 1 in]
            n532 = Build Array(w1081) -> (w1080:cluster{u32, u32}[])
            n533 = property on="DS 15" class="Bool (strict)"("Colors [4]"=w1080) -> ()  [unwired: 2 in, 2 out]
          }
          frame 15 {
            n534 = Bundle(w1082, w1082) -> (w1084:cluster{u32, u32})  [unwired: 1 in]
            n535 = Build Array(w1084) -> (w1083:cluster{u32, u32}[])
            n536 = property on="DS 16" class="Bool (strict)"("Colors [4]"=w1083) -> ()  [unwired: 2 in, 2 out]
          }
          frame 16 {
            n537 = Bundle(w1085, w1085) -> (w1087:cluster{u32, u32})  [unwired: 1 in]
            n538 = Build Array(w1087) -> (w1086:cluster{u32, u32}[])
            n539 = property on="DS 17" class="Bool (strict)"("Colors [4]"=w1086) -> ()  [unwired: 2 in, 2 out]
          }
          frame 17 {
            n540 = Bundle(w1088, w1088) -> (w1090:cluster{u32, u32})  [unwired: 1 in]
            n541 = Build Array(w1090) -> (w1089:cluster{u32, u32}[])
            n542 = property on="DS 18" class="Bool (strict)"("Colors [4]"=w1089) -> ()  [unwired: 2 in, 2 out]
          }
          frame 18 {
            n543 = Bundle(w1091, w1091) -> (w1093:cluster{u32, u32})  [unwired: 1 in]
            n544 = Build Array(w1093) -> (w1092:cluster{u32, u32}[])
            n545 = property on="DS 19" class="Bool (strict)"("Colors [4]"=w1092) -> ()  [unwired: 2 in, 2 out]
          }
          frame 19 {
            n546 = Bundle(w1094, w1094) -> (w1096:cluster{u32, u32})  [unwired: 1 in]
            n547 = Build Array(w1096) -> (w1095:cluster{u32, u32}[])
            n548 = property on="DS 20" class="Bool (strict)"("Colors [4]"=w1095) -> ()  [unwired: 2 in, 2 out]
          }
          frame 20 {
            n549 = Bundle(w1098, w1098) -> (w1100:cluster{u32, u32})  [unwired: 1 in]
            n550 = Build Array(w1100) -> (w1099:cluster{u32, u32}[])
            n551 = property on="DS 21" class="Bool (strict)"("Colors [4]"=w1099) -> (error out=w1097:errorcluster)  [unwired: 2 in, 1 out]
          }
        }
      }
    }
    frame Enabled {
    }
  }
  n552 = property class="App"(error in=w2) -> ("App.Kind"=w1:T7)  [unwired: 1 in, 2 out]
  n553 = case shown="\"Run Time System\"" w1 {
    frame "invalid app kind", Default {
    }
    frame "Development System" {
    }
    frame "Run Time System" {
      n554 = Quit LabVIEW() -> ()  [unwired: 1 in]
    }
    frame "Student Edition" {
    }
    frame "Embedded LabVIEW" {
    }
    frame "Evaluation" {
    }
    frame "Custom" {
    }
  }
